vi "Tool-Response Time.vi"() -> ()   [LabVIEW 2015]
uses:
  <vilib>/measure/mamon.llb/Trigger Detection for 1 Channel.vi
  <vilib>/measure/NI_MAPro.lvlib
panel:
  in  "hysteresis":dbl=0.4 format="%.2f"
  out "Cursor Info.":string="[cursor_raw]\n X: 32.346,  Y: 0.9937658\n\n[cursor_filter]\n X: 30.672,  Y: 0.9937830"
  in  "Exit":bool=TRUE
  in  "Calcuration":bool
  out "trigger detected? 2":bool=TRUE caption="트리거 검출?"
  out "trigger detected?":bool=TRUE caption="트리거 검출?"
  in  "Trigger level (%)":dbl=50.0 min=0.0 max=100.0
  out "Delay_time(s)":dbl=1.6739999999999782
  out "Delta-Filter":dbl=0.00020839999999999748
  out "Delta-Raw":dbl=0.00011250000000007088
  out "Data Length":i32=1387
  out "Response Time Graph":cluster{dbl[], dbl[]}[](graph)
  in  "Data in (Raw & Filter)":string="Time (H:M:S) - Left Wing-C\tCDC Ratio Data - Left Wing-C\tTime (H:M:S) - Right Wing-A\tCDC Ratio Data - Right Wing-A\n29:01.379\t0.9937134\t29:01.379\t0.9937296\n29:01.407\t0.9937134\t29:01.407\t0.9937143\n29:01.434\t0.9937134\t29:01.434\t0.9937077\n29:01.462\t0.9937139\t29:01.462\t0.9937186\n29:01.490\t0.9937139\t29:01.490\t0.9937115\n29:01.518\t0.9937134\t29:01.518\t0.9936929\n29:01.547\t0.9937134\t29:01.547\t0.9936919\n29:01.575\t0.9937134\t29:01.575\t0.9937086\n29:01.629\t0.9937129\t29:01.629\t0.9937015\n29:01.657\t0.9937124\t29:01.657\t0.9936986\n29:01.685\t0.9937124\t29:01.685\t0.9936953\n29:01.714\t0.9937124\t29:01.714\t0.9936929\n29:01.742\t0.9937124\t29:01.742\t0.9937029\n29:01.770\t0.9937124\t29:01.770\t0.9937029\n29:01.798\t0.9937124\t29:01.798\t0.9937181\n29:01.826\t0.9937124\t29:01.826\t0.9937124\n29:01.851\t0.9937124\t29:01.851\t0.9937172\n29:01.880\t0.9937129\t29:01.880\t0.9937143\n29:01.908\t0.9937129\t29:01.908\t0.9937038\n29:01.936\t0.9937129\t29:01.936\t0.993711\n29:01.993\t0.9937134\t29:01.993\t0.9937177\n29:02.021\t0.9937134\t29:02.021\t0.993711\n29:02.049\t0.9937139\t29:02.049\t0.9937196\n29:02.075\t0.9937139\t29:02.075\t0.9937091\n29:02.103\t0.9937139\t29:02.103\t0.9936996\n29:02.131\t0.9937139\t29:02.131\t0.9937124\n29:02.159\t0.9937143\t29:02.159\t0.9937325\n29:02.188\t0.9937148\t29:02.188\t0.9937649\n29:02.217\t0.9937153\t29:02.217\t0.9937749\n29:02.245\t0.9937162\t29:02.245\t0.9937549\n29:02.272\t0.9937167\t29:02.272\t0.9937334\n29:02.301\t0.9937167\t29:02.301\t0.9937248\n29:02.326\t0.9937167\t29:02.326\t0.993731\n29:02.383\t0.9937167\t29:02.383\t0.9937205\n29:02.411\t0.9937167\t29:02.411\t0.9937253\n29:02.439\t0.9937167\t29:02.439\t0.9937162\n29:02.467\t0.9937167\t29:02.467\t0.993752\n29:02.495\t0.9937172\t29:02.495\t0.9937534\n29:02.524\t0.9937177\t29:02.524\t0.9937453\n29:02.552\t0.9937181\t29:02.552\t0.9937339\n29:02.578\t0.9937186\t29:02.578\t0.9937229\n29:02.606\t0.9937186\t29:02.606\t0.9937358\n29:02.634\t0.9937191\t29:02.634\t0.9937229\n29:02.662\t0.9937191\t29:02.662\t0.9937229\n29:02.690\t0.9937191\t29:02.690\t0.99371\n29:02.719\t0.9937196\t29:02.719\t0.9937177\n29:02.746\t0.9937196\t29:02.746\t0.9937148\n29:02.800\t0.9937196\t29:02.800\t0.9937005\n29:02.828\t0.9937196\t29:02.828\t0.9937129\n29:02.856\t0.9937196\t29:02.856\t0.9937096\n29:02.884\t0.9937191\t29:02.884\t0.9937091\n29:02.913\t0.9937191\t29:02.913\t0.9937139\n29:02.941\t0.9937191\t29:02.941\t0.993711\n29:02.969\t0.9937186\t29:02.969\t0.9937096\n29:02.997\t0.9937181\t29:02.997\t0.9937139\n29:03.023\t0.9937181\t29:03.023\t0.9937115\n29:03.051\t0.9937181\t29:03.051\t0.9937291\n29:03.079\t0.9937181\t29:03.079\t0.9937205\n29:03.107\t0.9937181\t29:03.107\t0.9937215\n29:03.135\t0.9937177\t29:03.135\t0.9937215\n29:03.192\t0.9937177\t29:03.192\t0.9937048\n29:03.220\t0.9937177\t29:03.220\t0.9937034\n29:03.246\t0.9937181\t29:03.246\t0.9937143\n29:03.274\t0.9937181\t29:03.274\t0.9937062\n29:03.302\t0.9937181\t29:03.302\t0.9937143\n29:03.330\t0.9937177\t29:03.330\t0.9937215\n29:03.358\t0.9937177\t29:03.358\t0.9937115\n29:03.387\t0.9937177\t29:03.387\t0.9937158\n29:03.415\t0.9937177\t29:03.415\t0.9937129\n29:03.443\t0.9937177\t29:03.443\t0.9937119\n29:03.469\t0.9937172\t29:03.469\t0.9936972\n29:03.497\t0.9937172\t29:03.497\t0.9937191\n29:03.524\t0.9937172\t29:03.524\t0.9937143\n29:03.580\t0.9937172\t29:03.580\t0.9937081\n29:03.608\t0.9937172\t29:03.608\t0.9937201\n29:03.637\t0.9937172\t29:03.637\t0.9937119\n29:03.665\t0.9937177\t29:03.665\t0.9937205\n29:03.691\t0.9937177\t29:03.691\t0.9937263\n29:03.719\t0.9937177\t29:03.719\t0.9937286\n29:03.747\t0.9937177\t29:03.747\t0.9937148\n29:03.776\t0.9937177\t29:03.776\t0.9937086\n29:03.803\t0.9937177\t29:03.803\t0.9937119\n29:03.832\t0.9937177\t29:03.832\t0.9937191\n29:03.860\t0.9937177\t29:03.860\t0.9937072\n29:03.889\t0.9937177\t29:03.889\t0.9937062\n29:03.942\t0.9937177\t29:03.942\t0.9937305\n29:03.970\t0.9937177\t29:03.970\t0.9937258\n29:03.998\t0.9937177\t29:03.998\t0.9937167\n29:04.026\t0.9937177\t29:04.026\t0.9937081\n29:04.055\t0.9937177\t29:04.055\t0.9936981\n29:04.083\t0.9937177\t29:04.083\t0.9936967\n29:04.111\t0.9937172\t29:04.111\t0.9936976\n29:04.139\t0.9937172\t29:04.139\t0.993711\n29:04.165\t0.9937167\t29:04.165\t0.9937081\n29:04.193\t0.9937167\t29:04.193\t0.9937081\n29:04.221\t0.9937162\t29:04.221\t0.9937105\n29:04.250\t0.9937162\t29:04.250\t0.9937019\n29:04.278\t0.9937162\t29:04.278\t0.9937143\n29:04.306\t0.9937158\t29:04.306\t0.9937143\n29:04.362\t0.9937158\t29:04.362\t0.9936996\n29:04.388\t0.9937158\t29:04.388\t0.9937091\n29:04.416\t0.9937158\t29:04.416\t0.9937005\n29:04.444\t0.9937158\t29:04.444\t0.993721\n29:04.471\t0.9937162\t29:04.471\t0.9937358\n29:04.500\t0.9937167\t29:04.500\t0.9937267\n29:04.528\t0.9937167\t29:04.528\t0.9937253\n29:04.557\t0.9937172\t29:04.557\t0.9937258\n29:04.584\t0.9937172\t29:04.584\t0.9937234\n29:04.610\t0.9937177\t29:04.610\t0.9937077\n29:04.638\t0.9937177\t29:04.638\t0.9936996\n29:04.666\t0.9937172\t29:04.666\t0.9937\n29:04.695\t0.9937172\t29:04.695\t0.99369\n29:04.751\t0.9937167\t29:04.751\t0.9936943\n29:04.779\t0.9937167\t29:04.779\t0.9937\n29:04.807\t0.9937167\t29:04.807\t0.9937019\n29:04.833\t0.9937167\t29:04.833\t0.9937081\n29:04.861\t0.9937162\t29:04.861\t0.9937186\n29:04.889\t0.9937162\t29:04.889\t0.9937134\n29:04.918\t0.9937162\t29:04.918\t0.9937148\n29:04.946\t0.9937162\t29:04.946\t0.9937034\n29:04.974\t0.9937162\t29:04.974\t0.9937096\n29:05.002\t0.9937162\t29:05.002\t0.993721\n29:05.030\t0.9937162\t29:05.030\t0.9937263\n29:05.056\t0.9937162\t29:05.056\t0.9937272\n29:05.086\t0.9937162\t29:05.086\t0.9937425\n29:05.141\t0.9937158\t29:05.141\t0.993741\n29:05.169\t0.9937158\t29:05.169\t0.9937348\n29:05.197\t0.9937158\t29:05.197\t0.9937181\n29:05.225\t0.9937153\t29:05.225\t0.9937248\n29:05.254\t0.9937153\t29:05.254\t0.9937215\n29:05.279\t0.9937153\t29:05.279\t0.9937191\n29:05.307\t0.9937153\t29:05.307\t0.9937057\n29:05.335\t0.9937153\t29:05.335\t0.9937019\n29:05.364\t0.9937148\t29:05.364\t0.9937057\n29:05.392\t0.9937143\t29:05.392\t0.9936972\n29:05.420\t0.9937139\t29:05.420\t0.9937091\n29:05.447\t0.9937139\t29:05.447\t0.9937196\n29:05.476\t0.9937139\t29:05.476\t0.9937196\n29:05.529\t0.9937134\t29:05.529\t0.993722\n29:05.558\t0.9937134\t29:05.558\t0.9937091\n29:05.586\t0.9937134\t29:05.586\t0.9937148\n29:05.614\t0.9937134\t29:05.614\t0.9937296\n29:05.642\t0.9937134\t29:05.642\t0.9937162\n29:05.670\t0.9937134\t29:05.670\t0.9937143\n29:05.699\t0.9937134\t29:05.699\t0.9937124\n29:05.725\t0.9937134\t29:05.725\t0.9937148\n29:05.753\t0.9937134\t29:05.753\t0.9937115\n29:05.781\t0.9937134\t29:05.781\t0.9937081\n29:05.809\t0.9937134\t29:05.809\t0.9937096\n29:05.837\t0.9937134\t29:05.837\t0.9937139\n29:05.865\t0.9937134\t29:05.865\t0.9937186\n29:05.922\t0.9937139\t29:05.922\t0.9937162\n29:05.947\t0.9937139\t29:05.947\t0.9937229\n29:05.976\t0.9937134\t29:05.976\t0.9937034\n29:06.004\t0.9937134\t29:06.004\t0.99371\n29:06.032\t0.9937134\t29:06.032\t0.9937191\n29:06.060\t0.9937134\t29:06.060\t0.9937129\n29:06.088\t0.9937134\t29:06.088\t0.9937091\n29:06.117\t0.9937134\t29:06.117\t0.9937134\n29:06.145\t0.9937134\t29:06.145\t0.9937124\n29:06.173\t0.9937134\t29:06.173\t0.9937129\n29:06.199\t0.9937134\t29:06.199\t0.9937139\n29:06.227\t0.9937134\t29:06.227\t0.9937143\n29:06.254\t0.9937134\t29:06.254\t0.9937258\n29:06.311\t0.9937139\t29:06.311\t0.9937372\n29:06.339\t0.9937143\t29:06.339\t0.9937348\n29:06.368\t0.9937143\t29:06.368\t0.9937272\n29:06.396\t0.9937148\t29:06.396\t0.9937205\n29:06.421\t0.9937148\t29:06.421\t0.9937215\n29:06.449\t0.9937148\t29:06.449\t0.9937148\n29:06.477\t0.9937148\t29:06.477\t0.9937201\n29:06.505\t0.9937153\t29:06.505\t0.993731\n29:06.534\t0.9937153\t29:06.534\t0.9937167\n29:06.562\t0.9937153\t29:06.562\t0.9937057\n29:06.590\t0.9937153\t29:06.590\t0.9937181\n29:06.618\t0.9937148\t29:06.618\t0.9937158\n29:06.672\t0.9937148\t29:06.672\t0.9937129\n29:06.700\t0.9937148\t29:06.700\t0.9937105\n29:06.729\t0.9937148\t29:06.729\t0.9937077\n29:06.758\t0.9937148\t29:06.758\t0.9937067\n29:06.785\t0.9937148\t29:06.785\t0.9937086\n29:06.813\t0.9937148\t29:06.813\t0.9937057\n29:06.841\t0.9937148\t29:06.841\t0.9937239\n29:06.869\t0.9937143\t29:06.869\t0.993722\n29:06.895\t0.9937143\t29:06.895\t0.9937162\n29:06.923\t0.9937143\t29:06.923\t0.9937186\n29:06.951\t0.9937148\t29:06.951\t0.99371\n29:06.980\t0.9937148\t29:06.980\t0.9937253\n29:07.009\t0.9937148\t29:07.009\t0.9937282\n29:07.036\t0.9937153\t29:07.036\t0.9937105\n29:07.093\t0.9937148\t29:07.093\t0.99371\n29:07.118\t0.9937148\t29:07.118\t0.9936905\n29:07.147\t0.9937148\t29:07.147\t0.9936919\n29:07.175\t0.9937148\t29:07.175\t0.9936991\n29:07.203\t0.9937148\t29:07.203\t0.9937267\n29:07.230\t0.9937153\t29:07.230\t0.993763\n29:07.259\t0.9937158\t29:07.259\t0.9937725\n29:07.288\t0.9937162\t29:07.288\t0.9937325\n29:07.316\t0.9937167\t29:07.316\t0.9937167\n29:07.342\t0.9937167\t29:07.342\t0.9937167\n29:07.369\t0.9937162\t29:07.369\t0.9937201\n29:07.397\t0.9937162\t29:07.397\t0.9937234\n29:07.425\t0.9937162\t29:07.425\t0.9937253\n29:07.482\t0.9937162\t29:07.482\t0.9937224\n29:07.510\t0.9937162\t29:07.510\t0.9937363\n29:07.538\t0.9937167\t29:07.538\t0.9937496\n29:07.564\t0.9937172\t29:07.564\t0.9937444\n29:07.592\t0.9937177\t29:07.592\t0.9937158\n29:07.621\t0.9937177\t29:07.621\t0.993721\n29:07.650\t0.9937181\t29:07.650\t0.9937296\n29:07.677\t0.9937181\t29:07.677\t0.9937143\n29:07.705\t0.9937186\t29:07.705\t0.9937291\n29:07.733\t0.9937186\t29:07.733\t0.9937124\n29:07.761\t0.9937191\t29:07.761\t0.9937196\n29:07.790\t0.9937191\t29:07.790\t0.9937248\n29:07.816\t0.9937191\t29:07.816\t0.9937124\n29:07.872\t0.9937191\t29:07.872\t0.9937072\n29:07.900\t0.9937191\t29:07.900\t0.9937067\n29:07.928\t0.9937186\t29:07.928\t0.9937067\n29:07.957\t0.9937186\t29:07.957\t0.9937186\n29:07.985\t0.9937186\t29:07.985\t0.9937229\n29:08.013\t0.9937186\t29:08.013\t0.9937282\n29:08.039\t0.9937181\t29:08.039\t0.9937215\n29:08.067\t0.9937181\t29:08.067\t0.9937239\n29:08.095\t0.9937181\t29:08.095\t0.9937301\n29:08.123\t0.9937181\t29:08.123\t0.9937215\n29:08.152\t0.9937181\t29:08.152\t0.9937258\n29:08.179\t0.9937186\t29:08.179\t0.9937291\n29:08.207\t0.9937186\t29:08.207\t0.9937248\n29:08.235\t0.9937186\t29:08.235\t0.9937177\n29:08.289\t0.9937191\t29:08.289\t0.9937086\n29:08.317\t0.9937191\t29:08.317\t0.9936976\n29:08.346\t0.9937186\t29:08.346\t0.9937015\n29:08.374\t0.9937186\t29:08.374\t0.9936996\n29:08.402\t0.9937186\t29:08.402\t0.9936991\n29:08.430\t0.9937181\t29:08.430\t0.9936891\n29:08.459\t0.9937181\t29:08.459\t0.9936881\n29:08.487\t0.9937177\t29:08.487\t0.9936938\n29:08.513\t0.9937177\t29:08.513\t0.9936962\n29:08.541\t0.9937172\t29:08.541\t0.993711\n29:08.569\t0.9937172\t29:08.569\t0.9937086\n29:08.597\t0.9937172\t29:08.597\t0.9937005\n29:08.625\t0.9937172\t29:08.625\t0.9936967\n29:08.682\t0.9937172\t29:08.682\t0.9937\n29:08.710\t0.9937172\t29:08.710\t0.9937072\n29:08.736\t0.9937172\t29:08.736\t0.9937296\n29:08.764\t0.9937172\t29:08.764\t0.9937272\n29:08.792\t0.9937172\t29:08.792\t0.9937096\n29:08.820\t0.9937167\t29:08.820\t0.9937072\n29:08.848\t0.9937167\t29:08.848\t0.9936991\n29:08.876\t0.9937167\t29:08.876\t0.9937086\n29:08.905\t0.9937167\t29:08.905\t0.9936957\n29:08.935\t0.9937162\t29:08.935\t0.9936905\n29:08.959\t0.9937162\t29:08.959\t0.9936996\n29:08.987\t0.9937162\t29:08.987\t0.9937158\n29:09.014\t0.9937162\t29:09.014\t0.9937115\n29:09.071\t0.9937162\t29:09.071\t0.9937096\n29:09.100\t0.9937162\t29:09.100\t0.9937005\n29:09.128\t0.9937162\t29:09.128\t0.9937124\n29:09.156\t0.9937158\t29:09.156\t0.9937029\n29:09.182\t0.9937158\t29:09.182\t0.9937153\n29:09.209\t0.9937153\t29:09.209\t0.99371\n29:09.237\t0.9937153\t29:09.237\t0.9937091\n29:09.266\t0.9937148\t29:09.266\t0.9937067\n29:09.294\t0.9937148\t29:09.294\t0.9936981\n29:09.322\t0.9937143\t29:09.322\t0.9937143\n29:09.350\t0.9937143\t29:09.350\t0.9937038\n29:09.379\t0.9937143\t29:09.379\t0.9936948\n29:09.407\t0.9937139\t29:09.407\t0.9937048\n29:09.461\t0.9937139\t29:09.461\t0.9937086\n29:09.489\t0.9937139\t29:09.489\t0.9937286\n29:09.518\t0.9937139\t29:09.518\t0.9937358\n29:09.545\t0.9937143\t29:09.545\t0.9937272\n29:09.573\t0.9937143\t29:09.573\t0.9937305\n29:09.602\t0.9937148\t29:09.602\t0.993731\n29:09.630\t0.9937148\t29:09.630\t0.9937229\n29:09.656\t0.9937148\t29:09.656\t0.9937134\n29:09.684\t0.9937148\t29:09.684\t0.9937048\n29:09.712\t0.9937148\t29:09.712\t0.9937019\n29:09.740\t0.9937148\t29:09.740\t0.9937024\n29:09.769\t0.9937148\t29:09.769\t0.9937172\n29:09.797\t0.9937148\t29:09.797\t0.9937086\n29:09.824\t0.9937148\t29:09.824\t0.9937043\n29:09.879\t0.9937143\t29:09.879\t0.9937072\n29:09.906\t0.9937143\t29:09.906\t0.9937005\n29:09.934\t0.9937143\t29:09.934\t0.9937\n29:09.963\t0.9937139\t29:09.963\t0.9937048\n29:09.991\t0.9937139\t29:09.991\t0.9936962\n29:10.019\t0.9937139\t29:10.019\t0.9937067\n29:10.047\t0.9937143\t29:10.047\t0.9937196\n29:10.076\t0.9937143\t29:10.076\t0.9937305\n29:10.104\t0.9937148\t29:10.104\t0.9937291\n29:10.129\t0.9937143\t29:10.129\t0.9937334\n29:10.158\t0.9937143\t29:10.158\t0.9937344\n29:10.186\t0.9937139\t29:10.186\t0.9937305\n29:10.242\t0.9937139\t29:10.242\t0.9937129\n29:10.270\t0.9937139\t29:10.270\t0.9937205\n29:10.299\t0.9937139\t29:10.299\t0.9937267\n29:10.328\t0.9937143\t29:10.328\t0.9937286\n29:10.353\t0.9937139\t29:10.353\t0.9937072\n29:10.381\t0.9937139\t29:10.381\t0.9937038\n29:10.409\t0.9937134\t29:10.409\t0.9936914\n29:10.437\t0.9937129\t29:10.437\t0.9936924\n29:10.466\t0.9937124\t29:10.466\t0.9937029\n29:10.494\t0.9937124\t29:10.494\t0.9937267\n29:10.522\t0.9937124\t29:10.522\t0.9937129\n29:10.550\t0.9937124\t29:10.550\t0.9937062\n29:10.576\t0.9937124\t29:10.576\t0.9937077\n29:10.631\t0.9937119\t29:10.631\t0.9937077\n29:10.660\t0.9937119\t29:10.660\t0.9937282\n29:10.688\t0.9937119\t29:10.688\t0.993721\n29:10.716\t0.9937119\t29:10.716\t0.9937029\n29:10.744\t0.9937119\t29:10.744\t0.9937096\n29:10.772\t0.9937119\t29:10.772\t0.9937172\n29:10.798\t0.9937119\t29:10.798\t0.9937119\n29:10.827\t0.9937124\t29:10.827\t0.9937172\n29:10.854\t0.9937124\t29:10.854\t0.9937134\n29:10.882\t0.9937119\t29:10.882\t0.9937062\n29:10.911\t0.9937119\t29:10.911\t0.9937201\n29:10.939\t0.9937119\t29:10.939\t0.9937215\n29:10.967\t0.9937119\t29:10.967\t0.9937253\n29:10.995\t0.9937119\t29:10.995\t0.9937286\n29:11.049\t0.9937119\t29:11.049\t0.9937296\n29:11.077\t0.9937119\t29:11.077\t0.993732\n29:11.106\t0.9937119\t29:11.106\t0.9937243\n29:11.134\t0.9937119\t29:11.134\t0.9937067\n29:11.162\t0.9937119\t29:11.162\t0.9937124\n29:11.190\t0.9937119\t29:11.190\t0.9937119\n29:11.218\t0.9937119\t29:11.218\t0.9937167\n29:11.247\t0.9937119\t29:11.247\t0.9937139\n29:11.273\t0.9937119\t29:11.273\t0.9937215\n29:11.301\t0.9937124\t29:11.301\t0.9937191\n29:11.329\t0.9937124\t29:11.329\t0.9937348\n29:11.357\t0.9937134\t29:11.357\t0.9937363\n29:11.386\t0.9937134\t29:11.386\t0.9937282\n29:11.442\t0.9937139\t29:11.442\t0.9937181\n29:11.470\t0.9937143\t29:11.470\t0.9937229\n29:11.496\t0.9937143\t29:11.496\t0.9937067\n29:11.524\t0.9937143\t29:11.524\t0.993722\n29:11.553\t0.9937143\t29:11.553\t0.9937186\n29:11.581\t0.9937143\t29:11.581\t0.9937067\n29:11.609\t0.9937143\t29:11.609\t0.9936967\n29:11.637\t0.9937143\t29:11.637\t0.99371\n29:11.664\t0.9937143\t29:11.664\t0.9937129\n29:11.693\t0.9937143\t29:11.693\t0.9937053\n29:11.719\t0.9937143\t29:11.719\t0.9937077\n29:11.747\t0.9937139\t29:11.747\t0.9936962\n29:11.775\t0.9937139\t29:11.775\t0.9937005\n29:11.831\t0.9937143\t29:11.831\t0.9937153\n29:11.860\t0.9937143\t29:11.860\t0.99371\n29:11.888\t0.9937143\t29:11.888\t0.9937201\n29:11.916\t0.9937148\t29:11.916\t0.9937224\n29:11.944\t0.9937148\t29:11.944\t0.9937234\n29:11.970\t0.9937148\t29:11.970\t0.9937172\n29:11.999\t0.9937148\t29:11.999\t0.9937167\n29:12.026\t0.9937153\t29:12.026\t0.9937267\n29:12.054\t0.9937153\t29:12.054\t0.9937296\n29:12.083\t0.9937158\t29:12.083\t0.9937191\n29:12.112\t0.9937158\t29:12.112\t0.9937129\n29:12.140\t0.9937158\t29:12.140\t0.9937153\n29:12.167\t0.9937158\t29:12.167\t0.9936981\n29:12.221\t0.9937158\t29:12.221\t0.993722\n29:12.249\t0.9937158\t29:12.249\t0.9937487\n29:12.278\t0.9937162\t29:12.278\t0.9937663\n29:12.306\t0.9937172\t29:12.306\t0.993762\n29:12.334\t0.9937177\t29:12.334\t0.9937377\n29:12.362\t0.9937177\t29:12.362\t0.9937143\n29:12.390\t0.9937177\t29:12.390\t0.9937263\n29:12.419\t0.9937177\t29:12.419\t0.9937162\n29:12.444\t0.9937172\t29:12.444\t0.9937196\n29:12.473\t0.9937172\t29:12.473\t0.9937234\n29:12.501\t0.9937172\t29:12.501\t0.9937239\n29:12.529\t0.9937172\t29:12.529\t0.9937253\n29:12.558\t0.9937172\t29:12.558\t0.9937382\n29:12.613\t0.9937181\t29:12.613\t0.9937301\n29:12.641\t0.9937181\t29:12.641\t0.9937043\n29:12.667\t0.9937181\t29:12.667\t0.9937196\n29:12.695\t0.9937181\t29:12.695\t0.9937139\n29:12.723\t0.9937181\t29:12.723\t0.9937143\n29:12.751\t0.9937181\t29:12.751\t0.9937186\n29:12.779\t0.9937181\t29:12.779\t0.9937181\n29:12.807\t0.9937186\t29:12.807\t0.9937177\n29:12.835\t0.9937186\t29:12.835\t0.9937248\n29:12.864\t0.9937186\t29:12.864\t0.9937124\n29:12.890\t0.9937191\t29:12.890\t0.9937081\n29:12.918\t0.9937191\t29:12.918\t0.9937105\n29:12.946\t0.9937191\t29:12.946\t0.9937062\n29:13.002\t0.9937186\t29:13.002\t0.993722\n29:13.030\t0.9937186\t29:13.030\t0.9937229\n29:13.060\t0.9937186\t29:13.060\t0.9937263\n29:13.087\t0.9937186\t29:13.087\t0.9937215\n29:13.113\t0.9937181\t29:13.113\t0.9937277\n29:13.141\t0.9937186\t29:13.141\t0.9937224\n29:13.169\t0.9937186\t29:13.169\t0.9937253\n29:13.197\t0.9937186\t29:13.197\t0.993731\n29:13.225\t0.9937186\t29:13.225\t0.9937215\n29:13.253\t0.9937186\t29:13.253\t0.9937172\n29:13.282\t0.9937186\t29:13.282\t0.9937019\n29:13.310\t0.9937186\t29:13.310\t0.9937186\n29:13.336\t0.9937186\t29:13.336\t0.9937053\n29:13.392\t0.9937186\t29:13.392\t0.993722\n29:13.420\t0.9937186\t29:13.420\t0.9937024\n29:13.449\t0.9937186\t29:13.449\t0.9937024\n29:13.477\t0.9937186\t29:13.477\t0.9936938\n29:13.504\t0.9937181\t29:13.504\t0.993701\n29:13.532\t0.9937181\t29:13.532\t0.9936986\n29:13.560\t0.9937181\t29:13.560\t0.9937129\n29:13.586\t0.9937181\t29:13.586\t0.9937196\n29:13.614\t0.9937181\t29:13.614\t0.9937191\n29:13.643\t0.9937181\t29:13.643\t0.993701\n29:13.670\t0.9937181\t29:13.670\t0.9937148\n29:13.699\t0.9937181\t29:13.699\t0.9937158\n29:13.727\t0.9937181\t29:13.727\t0.9937057\n29:13.755\t0.9937181\t29:13.755\t0.9937072\n29:13.809\t0.9937181\t29:13.809\t0.9937201\n29:13.837\t0.9937181\t29:13.837\t0.9937196\n29:13.866\t0.9937181\t29:13.866\t0.9937115\n29:13.894\t0.9937181\t29:13.894\t0.9937196\n29:13.922\t0.9937181\t29:13.922\t0.9937072\n29:13.950\t0.9937177\t29:13.950\t0.9937034\n29:13.978\t0.9937177\t29:13.978\t0.9937096\n29:14.007\t0.9937172\t29:14.007\t0.9937124\n29:14.033\t0.9937172\t29:14.033\t0.9937148\n29:14.061\t0.9937172\t29:14.061\t0.9937153\n29:14.089\t0.9937172\t29:14.089\t0.9937015\n29:14.117\t0.9937172\t29:14.117\t0.9937015\n29:14.173\t0.9937167\t29:14.173\t0.9936895\n29:14.202\t0.9937167\t29:14.202\t0.9936986\n29:14.229\t0.9937162\t29:14.229\t0.9937015\n29:14.255\t0.9937158\t29:14.255\t0.993701\n29:14.283\t0.9937158\t29:14.283\t0.9936967\n29:14.311\t0.9937153\t29:14.311\t0.9936924\n29:14.340\t0.9937153\t29:14.340\t0.9937086\n29:14.368\t0.9937153\t29:14.368\t0.9937048\n29:14.396\t0.9937148\t29:14.396\t0.9937005\n29:14.424\t0.9937148\t29:14.424\t0.9936962\n29:14.453\t0.9937148\t29:14.453\t0.9936962\n29:14.481\t0.9937143\t29:14.481\t0.9936948\n29:14.508\t0.9937143\t29:14.508\t0.9937096\n29:14.535\t0.9937148\t29:14.535\t0.9937282\n29:14.591\t0.9937153\t29:14.591\t0.9937325\n29:14.619\t0.9937153\t29:14.619\t0.9937291\n29:14.647\t0.9937158\t29:14.647\t0.9937372\n29:14.675\t0.9937158\t29:14.675\t0.993731\n29:14.704\t0.9937162\t29:14.704\t0.9937201\n29:14.729\t0.9937162\t29:14.729\t0.99371\n29:14.758\t0.9937162\t29:14.758\t0.9937096\n29:14.786\t0.9937158\t29:14.786\t0.9937086\n29:14.814\t0.9937158\t29:14.814\t0.9937143\n29:14.842\t0.9937158\t29:14.842\t0.9937077\n29:14.870\t0.9937153\t29:14.870\t0.9937105\n29:14.898\t0.9937153\t29:14.898\t0.9937124\n29:14.926\t0.9937153\t29:14.926\t0.9937062\n29:14.981\t0.9937153\t29:14.981\t0.9937115\n29:15.009\t0.9937153\t29:15.009\t0.993701\n29:15.036\t0.9937148\t29:15.036\t0.9937081\n29:15.065\t0.9937153\t29:15.065\t0.993721\n29:15.092\t0.9937153\t29:15.092\t0.9937258\n29:15.121\t0.9937158\t29:15.121\t0.9937267\n29:15.149\t0.9937158\t29:15.149\t0.993742\n29:15.175\t0.9937153\t29:15.175\t0.993742\n29:15.203\t0.9937153\t29:15.203\t0.9937472\n29:15.231\t0.9937153\t29:15.231\t0.9937429\n29:15.259\t0.9937153\t29:15.259\t0.9937296\n29:15.287\t0.9937153\t29:15.287\t0.9937243\n29:15.316\t0.9937153\t29:15.316\t0.9937243\n29:15.372\t0.9937153\t29:15.372\t0.9937215\n29:15.398\t0.9937153\t29:15.398\t0.9937029\n29:15.426\t0.9937153\t29:15.426\t0.9937077\n29:15.454\t0.9937148\t29:15.454\t0.9936976\n29:15.483\t0.9937143\t29:15.483\t0.993701\n29:15.511\t0.9937139\t29:15.511\t0.9937158\n29:15.539\t0.9937143\t29:15.539\t0.9937358\n29:15.568\t0.9937143\t29:15.568\t0.9937191\n29:15.596\t0.9937143\t29:15.596\t0.9937224\n29:15.624\t0.9937143\t29:15.624\t0.9937067\n29:15.650\t0.9937143\t29:15.650\t0.993701\n29:15.678\t0.9937143\t29:15.678\t0.9937215\n29:15.706\t0.9937143\t29:15.706\t0.9937153\n29:15.762\t0.9937139\t29:15.762\t0.9937096\n29:15.791\t0.9937143\t29:15.791\t0.9937177\n29:15.819\t0.9937143\t29:15.819\t0.9937315\n29:15.847\t0.9937143\t29:15.847\t0.9937143\n29:15.872\t0.9937143\t29:15.872\t0.9937277\n29:15.900\t0.9937143\t29:15.900\t0.9937258\n29:15.929\t0.9937143\t29:15.929\t0.9937162\n29:15.957\t0.9937143\t29:15.957\t0.9937191\n29:15.986\t0.9937143\t29:15.986\t0.9937162\n29:16.013\t0.9937143\t29:16.013\t0.9937258\n29:16.042\t0.9937143\t29:16.042\t0.9937177\n29:16.070\t0.9937143\t29:16.070\t0.9937105\n29:16.098\t0.9937139\t29:16.098\t0.9937177\n29:16.152\t0.9937139\t29:16.152\t0.9937038\n29:16.180\t0.9937139\t29:16.180\t0.9937\n29:16.208\t0.9937134\t29:16.208\t0.9936943\n29:16.236\t0.9937134\t29:16.236\t0.9936934\n29:16.264\t0.9937134\t29:16.264\t0.993701\n29:16.292\t0.9937129\t29:16.292\t0.9936948\n29:16.321\t0.9937129\t29:16.321\t0.9937143\n29:16.348\t0.9937134\t29:16.348\t0.9937315\n29:16.376\t0.9937134\t29:16.376\t0.9937296\n29:16.403\t0.9937139\t29:16.403\t0.9937382\n29:16.431\t0.9937139\t29:16.431\t0.9937248\n29:16.460\t0.9937143\t29:16.460\t0.9937243\n29:16.488\t0.9937143\t29:16.488\t0.9937286\n29:16.516\t0.9937143\t29:16.516\t0.9937239\n29:16.570\t0.9937148\t29:16.570\t0.9937253\n29:16.598\t0.9937148\t29:16.598\t0.9937177\n29:16.628\t0.9937148\t29:16.628\t0.9937062\n29:16.654\t0.9937148\t29:16.654\t0.9937024\n29:16.683\t0.9937143\t29:16.683\t0.9937162\n29:16.710\t0.9937143\t29:16.710\t0.99371\n29:16.738\t0.9937143\t29:16.738\t0.9937158\n29:16.767\t0.9937143\t29:16.767\t0.9937096\n29:16.796\t0.9937143\t29:16.796\t0.9937029\n29:16.820\t0.9937139\t29:16.820\t0.9937115\n29:16.849\t0.9937143\t29:16.849\t0.9937148\n29:16.877\t0.9937143\t29:16.877\t0.9937077\n29:16.906\t0.9937143\t29:16.906\t0.9937105\n29:16.961\t0.9937143\t29:16.961\t0.9937229\n29:16.989\t0.9937143\t29:16.989\t0.9937191\n29:17.018\t0.9937143\t29:17.018\t0.9937038\n29:17.044\t0.9937143\t29:17.044\t0.9937177\n29:17.072\t0.9937148\t29:17.072\t0.9937239\n29:17.100\t0.9937148\t29:17.100\t0.9937201\n29:17.128\t0.9937153\t29:17.128\t0.9937072\n29:17.156\t0.9937153\t29:17.156\t0.9937143\n29:17.184\t0.9937153\t29:17.184\t0.9937139\n29:17.213\t0.9937153\t29:17.213\t0.9937005\n29:17.241\t0.9937158\t29:17.241\t0.9937124\n29:17.267\t0.9937158\t29:17.267\t0.9937315\n29:17.296\t0.9937162\t29:17.296\t0.9937806\n29:17.351\t0.9937177\t29:17.351\t0.9937696\n29:17.379\t0.9937181\t29:17.379\t0.9937415\n29:17.407\t0.9937186\t29:17.407\t0.9937425\n29:17.436\t0.9937186\t29:17.436\t0.9937353\n29:17.464\t0.9937186\t29:17.464\t0.9937239\n29:17.490\t0.9937186\t29:17.490\t0.9937267\n29:17.518\t0.9937186\t29:17.518\t0.9937267\n29:17.546\t0.9937186\t29:17.546\t0.9937162\n29:17.574\t0.9937186\t29:17.574\t0.9937401\n29:17.602\t0.9937186\t29:17.602\t0.9937449\n29:17.630\t0.9937191\t29:17.630\t0.9937372\n29:17.659\t0.9937196\t29:17.659\t0.9937277\n29:17.686\t0.9937196\t29:17.686\t0.9937129\n29:17.740\t0.9937196\t29:17.740\t0.9937124\n29:17.769\t0.9937196\t29:17.769\t0.9937191\n29:17.796\t0.9937196\t29:17.796\t0.9937096\n29:17.826\t0.9937196\t29:17.826\t0.9937153\n29:17.853\t0.9937196\t29:17.853\t0.9937162\n29:17.881\t0.9937196\t29:17.881\t0.9937186\n29:17.909\t0.9937196\t29:17.909\t0.9937015\n29:17.936\t0.9937196\t29:17.936\t0.9937081\n29:17.963\t0.9937196\t29:17.963\t0.9937105\n29:17.991\t0.9937196\t29:17.991\t0.9937053\n29:18.019\t0.9937191\t29:18.019\t0.9937153\n29:18.048\t0.9937191\t29:18.048\t0.9937148\n29:18.076\t0.9937186\t29:18.076\t0.9937134\n29:18.132\t0.9937181\t29:18.132\t0.9937167\n29:18.160\t0.9937181\t29:18.160\t0.9937296\n29:18.186\t0.9937181\t29:18.186\t0.9937124\n29:18.214\t0.9937181\t29:18.214\t0.9937239\n29:18.242\t0.9937181\t29:18.242\t0.9937239\n29:18.271\t0.9937181\t29:18.271\t0.9937153\n29:18.299\t0.9937181\t29:18.299\t0.99371\n29:18.327\t0.9937181\t29:18.327\t0.9937057\n29:18.356\t0.9937181\t29:18.356\t0.9937172\n29:18.384\t0.9937181\t29:18.384\t0.9937134\n29:18.409\t0.9937186\t29:18.409\t0.993731\n29:18.438\t0.9937186\t29:18.438\t0.9937348\n29:18.466\t0.9937181\t29:18.466\t0.9937148\n29:18.521\t0.9937181\t29:18.521\t0.9937224\n29:18.549\t0.9937186\t29:18.549\t0.9937258\n29:18.578\t0.9937186\t29:18.578\t0.9937234\n29:18.607\t0.9937186\t29:18.607\t0.9937353\n29:18.631\t0.9937191\t29:18.631\t0.9937468\n29:18.660\t0.9937191\t29:18.660\t0.9937444\n29:18.688\t0.9937196\t29:18.688\t0.9937272\n29:18.716\t0.9937196\t29:18.716\t0.9937482\n29:18.744\t0.9937201\t29:18.744\t0.993742\n29:18.773\t0.9937201\t29:18.773\t0.9937339\n29:18.801\t0.9937201\t29:18.801\t0.9937496\n29:18.829\t0.9937205\t29:18.829\t0.9937611\n29:18.856\t0.993721\t29:18.856\t0.9937544\n29:18.911\t0.9937215\t29:18.911\t0.9937372\n29:18.940\t0.9937215\t29:18.940\t0.993742\n29:18.968\t0.993722\t29:18.968\t0.9937329\n29:18.996\t0.993722\t29:18.996\t0.9937334\n29:19.024\t0.993722\t29:19.024\t0.993732\n29:19.052\t0.9937224\t29:19.052\t0.9937587\n29:19.081\t0.9937229\t29:19.081\t0.9937472\n29:19.107\t0.9937239\t29:19.107\t0.9937568\n29:19.135\t0.9937239\t29:19.135\t0.993751\n29:19.163\t0.9937243\t29:19.163\t0.9937482\n29:19.191\t0.9937248\t29:19.191\t0.993742\n29:19.219\t0.9937253\t29:19.219\t0.9937315\n29:19.249\t0.9937258\t29:19.249\t0.9937434\n29:19.276\t0.9937258\t29:19.276\t0.9937382\n29:19.329\t0.9937258\t29:19.329\t0.993731\n29:19.358\t0.9937258\t29:19.358\t0.9937296\n29:19.386\t0.9937258\t29:19.386\t0.9937296\n29:19.413\t0.9937258\t29:19.413\t0.9937334\n29:19.442\t0.9937263\t29:19.442\t0.9937329\n29:19.470\t0.9937263\t29:19.470\t0.9937382\n29:19.499\t0.9937263\t29:19.499\t0.9937444\n29:19.526\t0.9937267\t29:19.526\t0.9937401\n29:19.553\t0.9937272\t29:19.553\t0.9937644\n29:19.580\t0.9937277\t29:19.580\t0.9937806\n29:19.608\t0.9937282\t29:19.608\t0.9937768\n29:19.638\t0.9937291\t29:19.638\t0.9937701\n29:19.666\t0.9937296\t29:19.666\t0.9937634\n29:19.721\t0.9937305\t29:19.721\t0.9937572\n29:19.749\t0.993731\t29:19.749\t0.9937477\n29:19.776\t0.9937315\t29:19.776\t0.9937348\n29:19.804\t0.9937315\t29:19.804\t0.9937296\n29:19.832\t0.9937315\t29:19.832\t0.9937463\n29:19.860\t0.993732\t29:19.860\t0.9937458\n29:19.888\t0.9937325\t29:19.888\t0.9937468\n29:19.916\t0.9937325\t29:19.916\t0.9937477\n29:19.945\t0.9937329\t29:19.945\t0.9937544\n29:19.972\t0.9937334\t29:19.972\t0.9937596\n29:19.998\t0.9937339\t29:19.998\t0.9937592\n29:20.027\t0.9937344\t29:20.027\t0.993763\n29:20.055\t0.9937344\t29:20.055\t0.9937563\n29:20.111\t0.9937358\t29:20.111\t0.9937782\n29:20.139\t0.9937363\t29:20.139\t0.9937835\n29:20.168\t0.9937367\t29:20.168\t0.9937782\n29:20.196\t0.9937372\t29:20.196\t0.993782\n29:20.222\t0.9937372\t29:20.222\t0.9937825\n29:20.250\t0.9937372\t29:20.250\t0.9937863\n29:20.278\t0.9937377\t29:20.278\t0.9937873\n29:20.306\t0.9937377\t29:20.306\t0.9937625\n29:20.333\t0.9937382\t29:20.333\t0.9937701\n29:20.362\t0.9937387\t29:20.362\t0.9937744\n29:20.390\t0.9937391\t29:20.390\t0.993783\n29:20.419\t0.9937396\t29:20.419\t0.9937644\n29:20.448\t0.9937401\t29:20.448\t0.9937611\n29:20.501\t0.9937401\t29:20.501\t0.9937458\n29:20.528\t0.9937406\t29:20.528\t0.9937658\n29:20.558\t0.9937406\t29:20.558\t0.9937763\n29:20.586\t0.9937415\t29:20.586\t0.9937887\n29:20.613\t0.993742\t29:20.613\t0.9937792\n29:20.641\t0.9937425\t29:20.641\t0.9937706\n29:20.670\t0.9937429\t29:20.670\t0.9937592\n29:20.696\t0.9937434\t29:20.696\t0.9937673\n29:20.724\t0.9937439\t29:20.724\t0.993783\n29:20.752\t0.9937449\t29:20.752\t0.9937763\n29:20.780\t0.9937453\t29:20.780\t0.9937749\n29:20.808\t0.9937458\t29:20.808\t0.9937758\n29:20.837\t0.9937468\t29:20.837\t0.993782\n29:20.866\t0.9937472\t29:20.866\t0.9937825\n29:20.922\t0.9937487\t29:20.922\t0.9937735\n29:20.947\t0.9937491\t29:20.947\t0.9937673\n29:20.976\t0.9937496\t29:20.976\t0.9937758\n29:21.004\t0.9937501\t29:21.004\t0.9937854\n29:21.033\t0.993751\t29:21.033\t0.9937792\n29:21.060\t0.9937515\t29:21.060\t0.9937878\n29:21.088\t0.993752\t29:21.088\t0.9937797\n29:21.117\t0.9937525\t29:21.117\t0.9937773\n29:21.144\t0.9937534\t29:21.144\t0.9937797\n29:21.170\t0.9937539\t29:21.170\t0.9937763\n29:21.199\t0.9937544\t29:21.199\t0.9937663\n29:21.227\t0.9937549\t29:21.227\t0.9937654\n29:21.283\t0.9937558\t29:21.283\t0.9937677\n29:21.311\t0.9937563\t29:21.311\t0.9937744\n29:21.339\t0.9937568\t29:21.339\t0.9937725\n29:21.368\t0.9937572\t29:21.368\t0.993783\n29:21.396\t0.9937582\t29:21.396\t0.9937906\n29:21.421\t0.9937592\t29:21.421\t0.9938021\n29:21.450\t0.9937596\t29:21.450\t0.9938097\n29:21.478\t0.9937601\t29:21.478\t0.9937987\n29:21.506\t0.9937611\t29:21.506\t0.9937978\n29:21.534\t0.9937615\t29:21.534\t0.9938011\n29:21.562\t0.993762\t29:21.562\t0.9937887\n29:21.591\t0.993763\t29:21.591\t0.9938006\n29:21.619\t0.9937634\t29:21.619\t0.9938035\n29:21.646\t0.9937639\t29:21.646\t0.9937897\n29:21.701\t0.9937649\t29:21.701\t0.9937873\n29:21.731\t0.9937649\t29:21.731\t0.993794\n29:21.758\t0.9937654\t29:21.758\t0.993782\n29:21.786\t0.9937658\t29:21.786\t0.993783\n29:21.814\t0.9937663\t29:21.814\t0.9937778\n29:21.842\t0.9937663\t29:21.842\t0.9937692\n29:21.871\t0.9937668\t29:21.871\t0.9937901\n29:21.896\t0.9937677\t29:21.896\t0.9937892\n29:21.926\t0.9937677\t29:21.926\t0.9937797\n29:21.953\t0.9937682\t29:21.953\t0.9938025\n29:21.981\t0.9937687\t29:21.981\t0.993794\n29:22.009\t0.9937692\t29:22.009\t0.9938006\n29:22.039\t0.9937696\t29:22.039\t0.9937983\n29:22.066\t0.9937701\t29:22.066\t0.9937892\n29:22.120\t0.9937716\t29:22.120\t0.9938121\n29:22.148\t0.993772\t29:22.148\t0.9938002\n29:22.175\t0.9937725\t29:22.175\t0.9937906\n29:22.203\t0.9937735\t29:22.203\t0.9938064\n29:22.232\t0.9937739\t29:22.232\t0.993794\n29:22.260\t0.9937744\t29:22.260\t0.9937921\n29:22.289\t0.9937754\t29:22.289\t0.9937916\n29:22.316\t0.9937758\t29:22.316\t0.9938397\n29:22.346\t0.9937773\t29:22.346\t0.9938598\n29:22.371\t0.9937787\t29:22.371\t0.9938564\n29:22.399\t0.9937792\t29:22.399\t0.993835\n29:22.427\t0.9937801\t29:22.427\t0.9938121\n29:22.456\t0.9937806\t29:22.456\t0.9938154\n29:22.511\t0.9937811\t29:22.511\t0.9938092\n29:22.540\t0.9937816\t29:22.540\t0.9938068\n29:22.568\t0.993782\t29:22.568\t0.9938188\n29:22.594\t0.9937825\t29:22.594\t0.9938111\n29:22.622\t0.9937835\t29:22.622\t0.9938288\n29:22.650\t0.993784\t29:22.650\t0.9938426\n29:22.679\t0.9937849\t29:22.679\t0.993835\n29:22.707\t0.9937859\t29:22.707\t0.9938231\n29:22.736\t0.9937863\t29:22.736\t0.9938083\n29:22.763\t0.9937873\t29:22.763\t0.9938192\n29:22.791\t0.9937878\t29:22.791\t0.9938159\n29:22.820\t0.9937887\t29:22.820\t0.9938126\n29:22.846\t0.9937892\t29:22.846\t0.9938073\n29:22.903\t0.9937901\t29:22.903\t0.9938097\n29:22.930\t0.9937906\t29:22.930\t0.9938064\n29:22.958\t0.9937911\t29:22.958\t0.9937873\n29:22.987\t0.9937916\t29:22.987\t0.9937963\n29:23.015\t0.9937916\t29:23.015\t0.9937997\n29:23.043\t0.9937921\t29:23.043\t0.9938068\n29:23.069\t0.9937921\t29:23.069\t0.9938054\n29:23.097\t0.9937925\t29:23.097\t0.9938159\n29:23.124\t0.9937925\t29:23.124\t0.993814\n29:23.152\t0.993793\t29:23.152\t0.9938221\n29:23.181\t0.9937935\t29:23.181\t0.9938164\n29:23.209\t0.993794\t29:23.209\t0.9938202\n29:23.238\t0.9937944\t29:23.238\t0.9938188\n29:23.267\t0.9937949\t29:23.267\t0.9938207\n29:23.320\t0.9937959\t29:23.320\t0.9938159\n29:23.348\t0.9937963\t29:23.348\t0.9938064\n29:23.376\t0.9937963\t29:23.376\t0.9938116\n29:23.404\t0.9937973\t29:23.404\t0.9938092\n29:23.433\t0.9937978\t29:23.433\t0.9938097\n29:23.461\t0.9937983\t29:23.461\t0.9938159\n29:23.489\t0.9937983\t29:23.489\t0.9938068\n29:23.517\t0.9937987\t29:23.517\t0.9937954\n29:23.543\t0.9937987\t29:23.543\t0.993794\n29:23.571\t0.9937992\t29:23.571\t0.9938025\n29:23.600\t0.9937992\t29:23.600\t0.9938021\n29:23.628\t0.9937997\t29:23.628\t0.9937959\n29:23.656\t0.9938002\t29:23.656\t0.9938126\n29:23.712\t0.9938011\t29:23.712\t0.993814\n29:23.742\t0.9938016\t29:23.742\t0.9938221\n29:23.769\t0.9938016\t29:23.769\t0.9938188\n29:23.794\t0.9938021\t29:23.794\t0.9938064\n29:23.823\t0.9938025\t29:23.823\t0.9938231\n29:23.850\t0.993803\t29:23.850\t0.9938407\n29:23.878\t0.9938035\t29:23.878\t0.9938369\n29:23.906\t0.993804\t29:23.906\t0.9938226\n29:23.935\t0.9938045\t29:23.935\t0.9938126\n29:23.963\t0.9938049\t29:23.963\t0.9938207\n29:23.992\t0.9938049\t29:23.992\t0.9938154\n29:24.017\t0.9938054\t29:24.017\t0.9938035\n29:24.045\t0.9938054\t29:24.045\t0.9937983\n29:24.102\t0.9938059\t29:24.102\t0.9938235\n29:24.130\t0.9938068\t29:24.130\t0.9938188\n29:24.158\t0.9938068\t29:24.158\t0.9938054\n29:24.186\t0.9938073\t29:24.186\t0.9938059\n29:24.216\t0.9938078\t29:24.216\t0.9938006\n29:24.241\t0.9938083\t29:24.241\t0.9938073\n29:24.269\t0.9938083\t29:24.269\t0.9938097\n29:24.297\t0.9938087\t29:24.297\t0.9938178\n29:24.325\t0.9938087\t29:24.325\t0.9938207\n29:24.353\t0.9938087\t29:24.353\t0.9938159\n29:24.383\t0.9938087\t29:24.383\t0.9938045\n29:24.410\t0.9938092\t29:24.410\t0.9938164\n29:24.438\t0.9938092\t29:24.438\t0.9938111\n29:24.467\t0.9938092\t29:24.467\t0.9938083\n29:24.520\t0.9938092\t29:24.520\t0.9937959\n29:24.548\t0.9938092\t29:24.548\t0.9938021\n29:24.577\t0.9938097\t29:24.577\t0.9938006\n29:24.605\t0.9938097\t29:24.605\t0.9938211\n29:24.633\t0.9938102\t29:24.633\t0.9938288\n29:24.661\t0.9938107\t29:24.661\t0.9938192\n29:24.688\t0.9938107\t29:24.688\t0.9938211\n29:24.714\t0.9938111\t29:24.714\t0.9938273\n29:24.742\t0.9938116\t29:24.742\t0.9938269\n29:24.771\t0.9938121\t29:24.771\t0.9938068\n29:24.800\t0.9938121\t29:24.800\t0.9937997\n29:24.828\t0.9938126\t29:24.828\t0.9938054\n29:24.856\t0.9938126\t29:24.856\t0.9938016\n29:24.913\t0.9938126\t29:24.913\t0.9938126\n29:24.938\t0.993813\t29:24.938\t0.9938107\n29:24.966\t0.993813\t29:24.966\t0.9938111\n29:24.994\t0.993813\t29:24.994\t0.9938092\n29:25.022\t0.993813\t29:25.022\t0.9938059\n29:25.050\t0.993813\t29:25.050\t0.9938083\n29:25.079\t0.993813\t29:25.079\t0.9938068\n29:25.108\t0.993813\t29:25.108\t0.9938059\n29:25.136\t0.9938135\t29:25.136\t0.993824\n29:25.165\t0.993814\t29:25.165\t0.9938321\n29:25.189\t0.993814\t29:25.189\t0.9938264\n29:25.218\t0.9938145\t29:25.218\t0.9938359\n29:25.246\t0.993814\t29:25.246\t0.9938369\n29:25.302\t0.993814\t29:25.302\t0.9938388\n29:25.330\t0.993814\t29:25.330\t0.9938269\n29:25.358\t0.993814\t29:25.358\t0.9938145\n29:25.386\t0.993814\t29:25.386\t0.9938178\n29:25.412\t0.9938145\t29:25.412\t0.9938202\n29:25.441\t0.9938145\t29:25.441\t0.9938164\n29:25.469\t0.9938145\t29:25.469\t0.9938045\n29:25.498\t0.9938145\t29:25.498\t0.9938102\n29:25.525\t0.993814\t29:25.525\t0.9937987\n29:25.553\t0.9938135\t29:25.553\t0.9938087\n29:25.582\t0.9938135\t29:25.582\t0.9938107\n29:25.610\t0.9938135\t29:25.610\t0.9938374\n29:25.663\t0.9938135\t29:25.663\t0.9938283\n29:25.691\t0.9938135\t29:25.691\t0.9938259\n29:25.719\t0.9938135\t29:25.719\t0.9938135\n29:25.748\t0.993814\t29:25.748\t0.9938221\n29:25.775\t0.993814\t29:25.775\t0.9938226\n29:25.805\t0.993814\t29:25.805\t0.9938226\n29:25.833\t0.9938145\t29:25.833\t0.9938178\n29:25.860\t0.9938145\t29:25.860\t0.9938231\n29:25.886\t0.9938149\t29:25.886\t0.9938235\n29:25.914\t0.9938149\t29:25.914\t0.9938169\n29:25.942\t0.9938149\t29:25.942\t0.9938211\n29:25.971\t0.9938154\t29:25.971\t0.9938207\n29:26.000\t0.9938154\t29:26.000\t0.9938102\n29:26.027\t0.9938154\t29:26.027\t0.9938278\n29:26.055\t0.9938154\t29:26.055\t0.9938102\n29:26.109\t0.9938154\t29:26.109\t0.9938121\n29:26.137\t0.9938154\t29:26.137\t0.9938073\n29:26.166\t0.9938149\t29:26.166\t0.9938083\n29:26.194\t0.9938149\t29:26.194\t0.9938226\n29:26.222\t0.9938154\t29:26.222\t0.9938135\n29:26.251\t0.9938149\t29:26.251\t0.9938087\n29:26.278\t0.9938154\t29:26.278\t0.9938154\n29:26.307\t0.9938154\t29:26.307\t0.9938164\n29:26.333\t0.9938154\t29:26.333\t0.9938116\n29:26.361\t0.9938154\t29:26.361\t0.9938145\n29:26.389\t0.9938154\t29:26.389\t0.9938211\n29:26.417\t0.9938154\t29:26.417\t0.9938264\n29:26.472\t0.9938164\t29:26.472\t0.9938383\n29:26.502\t0.9938169\t29:26.502\t0.9938273\n29:26.529\t0.9938169\t29:26.529\t0.9938231\n29:26.555\t0.9938169\t29:26.555\t0.9938345\n29:26.584\t0.9938169\t29:26.584\t0.993824\n29:26.611\t0.9938169\t29:26.611\t0.9938154\n29:26.639\t0.9938173\t29:26.639\t0.9938321\n29:26.667\t0.9938173\t29:26.667\t0.993825\n29:26.696\t0.9938173\t29:26.696\t0.9938164\n29:26.724\t0.9938173\t29:26.724\t0.9938092\n29:26.752\t0.9938169\t29:26.752\t0.9938145\n29:26.781\t0.9938169\t29:26.781\t0.9938107\n29:26.806\t0.9938169\t29:26.806\t0.993814\n29:26.863\t0.9938164\t29:26.863\t0.9938064\n29:26.891\t0.9938164\t29:26.891\t0.9938149\n29:26.919\t0.9938164\t29:26.919\t0.9938164\n29:26.947\t0.9938169\t29:26.947\t0.9938111\n29:26.976\t0.9938169\t29:26.976\t0.9938188\n29:27.004\t0.9938169\t29:27.004\t0.9938183\n29:27.030\t0.9938169\t29:27.030\t0.9938331\n29:27.058\t0.9938169\t29:27.058\t0.9938269\n29:27.086\t0.9938173\t29:27.086\t0.9938207\n29:27.115\t0.9938173\t29:27.115\t0.9938107\n29:27.142\t0.9938173\t29:27.142\t0.9938307\n29:27.171\t0.9938178\t29:27.171\t0.9938226\n29:27.199\t0.9938178\t29:27.199\t0.9938107\n29:27.227\t0.9938178\t29:27.227\t0.9938116\n29:27.255\t0.9938173\t29:27.255\t0.9938126\n29:27.310\t0.9938173\t29:27.310\t0.9938049\n29:27.338\t0.9938173\t29:27.338\t0.9938183\n29:27.366\t0.9938178\t29:27.366\t0.9938564\n29:27.394\t0.9938183\t29:27.394\t0.9938922\n29:27.422\t0.9938192\t29:27.422\t0.9938664\n29:27.450\t0.9938197\t29:27.450\t0.9938383\n29:27.478\t0.9938202\t29:27.478\t0.9938378\n29:27.504\t0.9938202\t29:27.504\t0.9938374\n29:27.533\t0.9938207\t29:27.533\t0.9938254\n29:27.560\t0.9938207\t29:27.560\t0.9938307\n29:27.588\t0.9938207\t29:27.588\t0.9938207\n29:27.616\t0.9938207\t29:27.616\t0.9938154\n29:27.673\t0.9938207\t29:27.673\t0.9938474\n29:27.701\t0.9938211\t29:27.701\t0.9938502\n29:27.727\t0.9938216\t29:27.727\t0.9938369\n29:27.755\t0.9938216\t29:27.755\t0.9938083\n29:27.783\t0.9938216\t29:27.783\t0.9938221\n29:27.811\t0.9938221\t29:27.811\t0.9938202\n29:27.840\t0.9938221\t29:27.840\t0.9938192\n29:27.868\t0.9938221\t29:27.868\t0.9938059\n29:27.896\t0.9938221\t29:27.896\t0.9938116\n29:27.925\t0.9938221\t29:27.925\t0.9938149\n29:27.950\t0.9938221\t29:27.950\t0.9938178\n29:27.978\t0.9938221\t29:27.978\t0.9937935\n29:28.006\t0.9938221\t29:28.006\t0.9938002\n29:28.063\t0.9938216\t29:28.063\t0.9938092\n29:28.091\t0.9938216\t29:28.091\t0.9938188\n29:28.119\t0.9938216\t29:28.119\t0.9938245\n29:28.147\t0.9938211\t29:28.147\t0.9938149\n29:28.174\t0.9938211\t29:28.174\t0.9938197\n29:28.200\t0.9938211\t29:28.200\t0.9938216\n29:28.229\t0.9938211\t29:28.229\t0.9938264\n29:28.258\t0.9938211\t29:28.258\t0.9938312\n29:28.285\t0.9938211\t29:28.285\t0.9938354\n29:28.313\t0.9938211\t29:28.313\t0.9938312\n29:28.341\t0.9938211\t29:28.341\t0.9938226\n29:28.369\t0.9938211\t29:28.369\t0.9938087\n29:28.399\t0.9938211\t29:28.399\t0.993804\n29:28.452\t0.9938216\t29:28.452\t0.9938102\n29:28.480\t0.9938216\t29:28.480\t0.993813\n29:28.508\t0.9938216\t29:28.508\t0.9938259\n29:28.536\t0.9938216\t29:28.536\t0.9938073\n29:28.565\t0.9938211\t29:28.565\t0.993814\n29:28.593\t0.9938211\t29:28.593\t0.9938045\n29:28.621\t0.9938211\t29:28.621\t0.993804\n29:28.647\t0.9938207\t29:28.647\t0.9938049\n29:28.675\t0.9938207\t29:28.675\t0.9938169\n29:28.703\t0.9938207\t29:28.703\t0.9938154\n29:28.733\t0.9938207\t29:28.733\t0.993825\n29:28.760\t0.9938207\t29:28.760\t0.9938083\n29:28.788\t0.9938207\t29:28.788\t0.993825\n29:28.816\t0.9938207\t29:28.816\t0.9938188\n29:28.873\t0.9938202\t29:28.873\t0.993824\n29:28.898\t0.9938207\t29:28.898\t0.9938293\n29:28.927\t0.9938207\t29:28.927\t0.9938245\n29:28.955\t0.9938207\t29:28.955\t0.9938202\n29:28.984\t0.9938207\t29:28.984\t0.9938135\n29:29.011\t0.9938207\t29:29.011\t0.9938178\n29:29.039\t0.9938207\t29:29.039\t0.9938097\n29:29.068\t0.9938207\t29:29.068\t0.9938073\n29:29.097\t0.9938207\t29:29.097\t0.9938083\n29:29.122\t0.9938207\t29:29.122\t0.993824\n29:29.150\t0.9938207\t29:29.150\t0.9938202\n29:29.177\t0.9938207\t29:29.177\t0.9938126\n29:29.206\t0.9938207\t29:29.206\t0.9938107\n29:29.262\t0.9938207\t29:29.262\t0.9938073\n29:29.290\t0.9938202\t29:29.290\t0.9938025\n29:29.318\t0.9938202\t29:29.318\t0.9938092\n29:29.344\t0.9938197\t29:29.344\t0.9938021\n29:29.372\t0.9938197\t29:29.372\t0.993803\n29:29.400\t0.9938192\t29:29.400\t0.9938102\n29:29.428\t0.9938192\t29:29.428\t0.9938054\n29:29.457\t0.9938188\t29:29.457\t0.9937963\n29:29.485\t0.9938188\t29:29.485\t0.9938107\n29:29.513\t0.9938188\t29:29.513\t0.9938016\n29:29.541\t0.9938183\t29:29.541\t0.9938002\n29:29.567\t0.9938178\t29:29.567\t0.9938145\n29:29.595\t0.9938178\t29:29.595\t0.9938059\n29:29.651\t0.9938183\t29:29.651\t0.9938354\n29:29.679\t0.9938183\t29:29.679\t0.9938378\n29:29.708\t0.9938188\t29:29.708\t0.993835\n29:29.736\t0.9938188\t29:29.736\t0.9938321\n29:29.764\t0.9938188\t29:29.764\t0.993825\n29:29.794\t0.9938192\t29:29.794\t0.9938197\n29:29.819\t0.9938188\t29:29.819\t0.9938049\n29:29.848\t0.9938188\t29:29.848\t0.9938045\n29:29.875\t0.9938188\t29:29.875\t0.9937983\n29:29.903\t0.9938188\t29:29.903\t0.9938116\n29:29.931\t0.9938183\t29:29.931\t0.9938126\n29:29.960\t0.9938183\t29:29.960\t0.9938197\n29:29.988\t0.9938183\t29:29.988\t0.9938159\n29:30.016\t0.9938183\t29:30.016\t0.9938207\n29:30.070\t0.9938183\t29:30.070\t0.9938231\n29:30.097\t0.9938183\t29:30.097\t0.993824\n29:30.126\t0.9938183\t29:30.126\t0.9938169\n29:30.154\t0.9938183\t29:30.154\t0.9938135\n29:30.183\t0.9938188\t29:30.183\t0.9938397\n29:30.210\t0.9938192\t29:30.210\t0.9938455\n29:30.238\t0.9938192\t29:30.238\t0.9938412\n29:30.265\t0.9938192\t29:30.265\t0.9938488\n29:30.292\t0.9938192\t29:30.292\t0.9938483\n29:30.321\t0.9938188\t29:30.321\t0.9938431\n29:30.350\t0.9938188\t29:30.350\t0.9938431\n29:30.377\t0.9938188\t29:30.377\t0.9938188\n29:30.406\t0.9938183\t29:30.406\t0.9938297\n29:30.462\t0.9938183\t29:30.462\t0.993824\n29:30.490\t0.9938183\t29:30.490\t0.9938173\n29:30.516\t0.9938183\t29:30.516\t0.9938126\n29:30.545\t0.9938178\t29:30.545\t0.9938054\n29:30.572\t0.9938178\t29:30.572\t0.9938006\n29:30.601\t0.9938173\t29:30.601\t0.9938135\n29:30.629\t0.9938169\t29:30.629\t0.9938269\n29:30.657\t0.9938173\t29:30.657\t0.9938369\n29:30.685\t0.9938173\t29:30.685\t0.993824\n29:30.715\t0.9938173\t29:30.715\t0.9938197\n29:30.739\t0.9938173\t29:30.739\t0.993804\n29:30.768\t0.9938169\t29:30.768\t0.9938097\n29:30.796\t0.9938173\t29:30.796\t0.9938207\n29:30.851\t0.9938173\t29:30.851\t0.9938145\n29:30.880\t0.9938173\t29:30.880\t0.9938188\n29:30.908\t0.9938178\t29:30.908\t0.9938169\n29:30.936\t0.9938178\t29:30.936\t0.9938254\n29:30.964\t0.9938178\t29:30.964\t0.9938169\n29:30.990\t0.9938178\t29:30.990\t0.9938259\n29:31.018\t0.9938178\t29:31.018\t0.9938173\n29:31.046\t0.9938178\t29:31.046\t0.9938192\n29:31.075\t0.9938178\t29:31.075\t0.9938321\n29:31.103\t0.9938178\t29:31.103\t0.9938211\n29:31.132\t0.9938178\t29:31.132\t0.9938235\n29:31.159\t0.9938178\t29:31.159\t0.9938231\n29:31.187\t0.9938178\t29:31.187\t0.9938154\n29:31.241\t0.9938178\t29:31.241\t0.9938145\n29:31.269\t0.9938178\t29:31.269\t0.9938107\n29:31.298\t0.9938178\t29:31.298\t0.9938087\n29:31.326\t0.9938178\t29:31.326\t0.9938159\n29:31.355\t0.9938178\t29:31.355\t0.9938078\n29:31.382\t0.9938178\t29:31.382\t0.9938154\n29:31.411\t0.9938178\t29:31.411\t0.9938149\n29:31.436\t0.9938178\t29:31.436\t0.993825\n29:31.465\t0.9938178\t29:31.465\t0.9938426\n29:31.493\t0.9938183\t29:31.493\t0.9938383\n29:31.521\t0.9938188\t29:31.521\t0.9938512\n29:31.549\t0.9938188\t29:31.549\t0.9938345\n29:31.578\t0.9938192\t29:31.578\t0.993834\n29:31.607\t0.9938192\t29:31.607\t0.9938345\n29:31.662\t0.9938197\t29:31.662\t0.9938273\n29:31.688\t0.9938197\t29:31.688\t0.9938378\n29:31.715\t0.9938197\t29:31.715\t0.9938259\n29:31.744\t0.9938197\t29:31.744\t0.9938068\n29:31.772\t0.9938197\t29:31.772\t0.9938116\n29:31.800\t0.9938197\t29:31.800\t0.9938154\n29:31.828\t0.9938192\t29:31.828\t0.9938049\n29:31.857\t0.9938192\t29:31.857\t0.9938092\n29:31.885\t0.9938192\t29:31.885\t0.9938073\n29:31.910\t0.9938188\t29:31.910\t0.9938083\n29:31.938\t0.9938192\t29:31.938\t0.9938254\n29:31.967\t0.9938192\t29:31.967\t0.9938178\n29:31.995\t0.9938192\t29:31.995\t0.9937973\n29:32.051\t0.9938188\t29:32.051\t0.993783\n29:32.079\t0.9938183\t29:32.079\t0.9937782\n29:32.108\t0.9938178\t29:32.108\t0.9937596\n29:32.134\t0.9938173\t29:32.134\t0.9937472\n29:32.162\t0.9938169\t29:32.162\t0.9937611\n29:32.190\t0.9938169\t29:32.190\t0.9937525\n29:32.218\t0.9938159\t29:32.218\t0.9937434\n29:32.246\t0.9938154\t29:32.246\t0.9937224\n29:32.275\t0.9938145\t29:32.275\t0.9937325\n29:32.303\t0.9938135\t29:32.303\t0.9937229\n29:32.331\t0.9938126\t29:32.331\t0.9937072\n29:32.359\t0.9938121\t29:32.359\t0.993711\n29:32.385\t0.9938111\t29:32.385\t0.9937444\n29:32.441\t0.9938107\t29:32.441\t0.9937768\n29:32.469\t0.9938102\t29:32.469\t0.9937558\n29:32.498\t0.9938097\t29:32.498\t0.9937367\n29:32.526\t0.9938087\t29:32.526\t0.9937325\n29:32.554\t0.9938078\t29:32.554\t0.9937329\n29:32.583\t0.9938068\t29:32.583\t0.9937277\n29:32.608\t0.9938054\t29:32.608\t0.9937253\n29:32.636\t0.9938045\t29:32.636\t0.9937353\n29:32.665\t0.993804\t29:32.665\t0.99371\n29:32.693\t0.993803\t29:32.693\t0.993741\n29:32.721\t0.9938021\t29:32.721\t0.9937472\n29:32.749\t0.9938016\t29:32.749\t0.9937348\n29:32.777\t0.9938011\t29:32.777\t0.9937286\n29:32.805\t0.9938002\t29:32.805\t0.993722\n29:32.859\t0.9937983\t29:32.859\t0.9937215\n29:32.887\t0.9937978\t29:32.887\t0.9937172\n29:32.916\t0.9937968\t29:32.916\t0.9937205\n29:32.943\t0.9937959\t29:32.943\t0.9937234\n29:32.972\t0.9937949\t29:32.972\t0.993722\n29:33.000\t0.993794\t29:33.000\t0.993721\n29:33.028\t0.9937925\t29:33.028\t0.9937005\n29:33.056\t0.9937916\t29:33.056\t0.9937143\n29:33.082\t0.9937906\t29:33.082\t0.9937105\n29:33.110\t0.9937897\t29:33.110\t0.993711\n29:33.138\t0.9937882\t29:33.138\t0.9937096\n29:33.168\t0.9937873\t29:33.168\t0.9937177\n29:33.195\t0.9937859\t29:33.195\t0.9937129\n29:33.251\t0.9937835\t29:33.251\t0.9937201\n29:33.280\t0.9937825\t29:33.280\t0.9937229\n29:33.305\t0.9937816\t29:33.305\t0.993721\n29:33.334\t0.9937806\t29:33.334\t0.9937263\n29:33.362\t0.9937797\t29:33.362\t0.9937248\n29:33.390\t0.9937787\t29:33.390\t0.9937267\n29:33.418\t0.9937778\t29:33.418\t0.9937086\n29:33.447\t0.9937768\t29:33.447\t0.9937148\n29:33.475\t0.9937758\t29:33.475\t0.9937129\n29:33.503\t0.9937749\t29:33.503\t0.9937048\n29:33.531\t0.9937739\t29:33.531\t0.99371\n29:33.557\t0.9937725\t29:33.557\t0.9937086\n29:33.613\t0.9937706\t29:33.613\t0.9937015\n29:33.641\t0.9937696\t29:33.641\t0.9936957\n29:33.669\t0.9937682\t29:33.669\t0.9936976\n29:33.697\t0.9937673\t29:33.697\t0.9936919\n29:33.725\t0.9937658\t29:33.725\t0.993711\n29:33.754\t0.9937649\t29:33.754\t0.993722\n29:33.780\t0.9937639\t29:33.780\t0.9936976\n29:33.808\t0.9937625\t29:33.808\t0.9937\n29:33.836\t0.993762\t29:33.836\t0.9937124\n29:33.865\t0.9937606\t29:33.865\t0.9937\n29:33.892\t0.9937596\t29:33.892\t0.9937077\n29:33.921\t0.9937582\t29:33.921\t0.9937172\n29:33.949\t0.9937572\t29:33.949\t0.9937196\n29:33.978\t0.9937563\t29:33.978\t0.9937057\n29:34.005\t0.9937549\t29:34.005\t0.9937077\n29:34.059\t0.9937525\t29:34.059\t0.9937096\n29:34.088\t0.993752\t29:34.088\t0.9937053\n29:34.116\t0.9937506\t29:34.116\t0.9936986\n29:34.144\t0.9937496\t29:34.144\t0.9937005\n29:34.172\t0.9937487\t29:34.172\t0.9937234\n29:34.200\t0.9937477\t29:34.200\t0.9937139\n29:34.229\t0.9937463\t29:34.229\t0.9936986\n29:34.255\t0.9937453\t29:34.255\t0.9937015\n29:34.283\t0.9937439\t29:34.283\t0.9936924\n29:34.312\t0.9937434\t29:34.312\t0.9936962\n29:34.339\t0.993742\t29:34.339\t0.9936857\n29:34.367\t0.993741\t29:34.367\t0.9937086\n29:34.394\t0.9937396\t29:34.394\t0.9937038\n29:34.451\t0.9937363\t29:34.451\t0.9936957\n29:34.477\t0.9937348\t29:34.477\t0.9936948\n29:34.505\t0.9937339\t29:34.505\t0.9937043\n29:34.533\t0.9937329\t29:34.533\t0.9936962\n29:34.561\t0.9937315\t29:34.561\t0.9936838\n29:34.589\t0.9937301\t29:34.589\t0.9936905\n29:34.618\t0.9937286\t29:34.618\t0.9936996\n29:34.646\t0.9937277\t29:34.646\t0.9937019\n29:34.674\t0.9937267\t29:34.674\t0.9937272\n29:34.700\t0.9937258\t29:34.700\t0.9937334\n29:34.728\t0.9937248\t29:34.728\t0.9937201\n29:34.756\t0.9937243\t29:34.756\t0.9937248\n29:34.812\t0.9937224\t29:34.812\t0.9937272\n29:34.841\t0.9937215\t29:34.841\t0.993711\n29:34.869\t0.9937205\t29:34.869\t0.9936948\n29:34.897\t0.9937191\t29:34.897\t0.9936962\n29:34.923\t0.9937181\t29:34.923\t0.993691\n29:34.951\t0.9937172\t29:34.951\t0.9936972\n29:34.981\t0.9937167\t29:34.981\t0.9936962\n29:35.008\t0.9937158\t29:35.008\t0.9937038\n29:35.036\t0.9937153\t29:35.036\t0.9937053\n29:35.064\t0.9937148\t29:35.064\t0.9937072\n29:35.092\t0.9937143\t29:35.092\t0.9937162\n29:35.120\t0.9937139\t29:35.120\t0.9937038\n29:35.147\t0.9937139\t29:35.147\t0.9936996\n29:35.203\t0.9937134\t29:35.203\t0.9937043\n29:35.231\t0.9937134\t29:35.231\t0.9937296\n29:35.259\t0.9937139\t29:35.259\t0.993732\n29:35.288\t0.9937139\t29:35.288\t0.9937267\n29:35.315\t0.9937134\t29:35.315\t0.9937387\n29:35.343\t0.9937129\t29:35.343\t0.9937377\n29:35.372\t0.9937129\t29:35.372\t0.993731\n29:35.397\t0.9937124\t29:35.397\t0.9937243\n29:35.425\t0.9937124\t29:35.425\t0.9937096\n29:35.453\t0.9937124\t29:35.453\t0.9937139\n29:35.481\t0.9937119\t29:35.481\t0.9937186\n29:35.509\t0.9937119\t29:35.509\t0.9937124\n29:35.538\t0.9937119\t29:35.538\t0.9937048\n29:35.566\t0.9937119\t29:35.566\t0.9937053\n29:35.620\t0.993711\t29:35.620\t0.9937053\n29:35.649\t0.9937105\t29:35.649\t0.9937096\n29:35.676\t0.9937105\t29:35.676\t0.9937282\n29:35.704\t0.9937105\t29:35.704\t0.9937229\n29:35.733\t0.9937105\t29:35.733\t0.9937196\n29:35.761\t0.9937105\t29:35.761\t0.993722\n29:35.789\t0.9937105\t29:35.789\t0.9937057\n29:35.817\t0.9937105\t29:35.817\t0.9937158\n29:35.843\t0.9937105\t29:35.843\t0.993721\n29:35.871\t0.9937105\t29:35.871\t0.9937181\n29:35.900\t0.99371\t29:35.900\t0.9937167\n29:35.928\t0.99371\t29:35.928\t0.9937181\n29:35.956\t0.9937105\t29:35.956\t0.9937186\n29:36.012\t0.99371\t29:36.012\t0.9937086\n29:36.040\t0.99371\t29:36.040\t0.9937091\n29:36.066\t0.99371\t29:36.066\t0.9937024\n29:36.094\t0.99371\t29:36.094\t0.993722\n29:36.123\t0.99371\t29:36.123\t0.9937339\n29:36.152\t0.9937105\t29:36.152\t0.9937215\n29:36.179\t0.99371\t29:36.179\t0.9937267\n29:36.207\t0.99371\t29:36.207\t0.9937129\n29:36.235\t0.99371\t29:36.235\t0.9937134\n29:36.264\t0.99371\t29:36.264\t0.9937239\n29:36.292\t0.99371\t29:36.292\t0.9937191\n29:36.317\t0.9937096\t29:36.317\t0.9937081\n29:36.345\t0.9937096\t29:36.345\t0.9937081\n29:36.401\t0.9937096\t29:36.401\t0.9937115\n29:36.429\t0.9937096\t29:36.429\t0.9937134\n29:36.458\t0.9937096\t29:36.458\t0.9937224\n29:36.486\t0.99371\t29:36.486\t0.9937215\n29:36.515\t0.99371\t29:36.515\t0.9937329\n29:36.540\t0.9937105\t29:36.540\t0.9937401\n29:36.568\t0.993711\t29:36.568\t0.9937334\n29:36.597\t0.9937115\t29:36.597\t0.9937344\n29:36.625\t0.9937115\t29:36.625\t0.9937248\n29:36.653\t0.9937119\t29:36.653\t0.9937243\n29:36.681\t0.9937119\t29:36.681\t0.9937153\n29:36.709\t0.9937124\t29:36.709\t0.9937305\n29:36.737\t0.9937124\t29:36.737\t0.9937229\n29:36.791\t0.9937124\t29:36.791\t0.9937105\n29:36.819\t0.9937124\t29:36.819\t0.9937153\n29:36.849\t0.9937124\t29:36.849\t0.9937115\n29:36.876\t0.9937124\t29:36.876\t0.9936991\n29:36.904\t0.9937124\t29:36.904\t0.9936996\n29:36.933\t0.9937124\t29:36.933\t0.9936996\n29:36.960\t0.9937124\t29:36.960\t0.9937048\n29:36.986\t0.9937124\t29:36.986\t0.99371\n29:37.015\t0.9937124\t29:37.015\t0.9937105\n29:37.042\t0.9937124\t29:37.042\t0.9937077\n29:37.071\t0.9937124\t29:37.071\t0.9937224\n29:37.099\t0.9937124\t29:37.099\t0.9937229\n29:37.126\t0.9937129\t29:37.126\t0.9937129\n29:37.182\t0.9937129\t29:37.182\t0.9937086\n29:37.208\t0.9937134\t29:37.208\t0.9937277\n29:37.236\t0.9937134\t29:37.236\t0.9937239\n29:37.265\t0.9937139\t29:37.265\t0.9937282\n29:37.293\t0.9937139\t29:37.293\t0.9937172\n29:37.321\t0.9937139\t29:37.321\t0.9937191\n29:37.349\t0.9937143\t29:37.349\t0.9937024\n29:37.377\t0.9937143\t29:37.377\t0.9937062\n29:37.406\t0.9937143\t29:37.406\t0.9937186\n29:37.434\t0.9937148\t29:37.434\t0.9937572\n29:37.460\t0.9937158\t29:37.460\t0.9937901\n29:37.488\t0.9937167\t29:37.488\t0.9937644\n29:37.516\t0.9937172\t29:37.516\t0.9937544\n29:37.572\t0.9937177\t29:37.572\t0.9937329\n29:37.601\t0.9937177\t29:37.601\t0.993732\n29:37.629\t0.9937177\t29:37.629\t0.993731\n29:37.657\t0.9937177\t29:37.657\t0.9937282\n29:37.685\t0.9937181\t29:37.685\t0.9937296\n29:37.711\t0.9937181\t29:37.711\t0.9937377\n29:37.739\t0.9937181\t29:37.739\t0.993742\n29:37.768\t0.9937186\t29:37.768\t0.9937534\n29:37.796\t0.9937191\t29:37.796\t0.9937525\n29:37.823\t0.9937196\t29:37.823\t0.9937272\n29:37.853\t0.9937201\t29:37.853\t0.9937267\n29:37.881\t0.9937201\t29:37.881\t0.993722\n29:37.908\t0.9937205\t29:37.908\t0.9937162\n29:37.962\t0.9937205\t29:37.962\t0.993711\n29:37.990\t0.9937205\t29:37.990\t0.99371\n29:38.018\t0.9937205\t29:38.018\t0.9937162\n29:38.046\t0.993721\t29:38.046\t0.9937119\n29:38.075\t0.993721\t29:38.075\t0.9937038\n29:38.103\t0.993721\t29:38.103\t0.9937181\n29:38.131\t0.993721\t29:38.131\t0.9937124\n29:38.159\t0.9937205\t29:38.159\t0.9937148\n29:38.185\t0.9937205\t29:38.185\t0.9937243\n29:38.214\t0.9937205\t29:38.214\t0.9937286\n29:38.242\t0.9937205\t29:38.242\t0.993731\n29:38.270\t0.9937205\t29:38.270\t0.9937196\n29:38.298\t0.9937205\t29:38.298\t0.9937339\n29:38.326\t0.9937205\t29:38.326\t0.9937387\n29:38.355\t0.9937205\t29:38.355\t0.9937387\n29:38.411\t0.993721\t29:38.411\t0.9937325\n29:38.437\t0.993721\t29:38.437\t0.9937234\n29:38.465\t0.9937215\t29:38.465\t0.9937215\n29:38.493\t0.9937215\t29:38.493\t0.9937196\n29:38.521\t0.9937215\t29:38.521\t0.9937191\n29:38.550\t0.993722\t29:38.550\t0.9937081\n29:38.579\t0.9937215\t29:38.579\t0.9937215\n29:38.606\t0.9937215\t29:38.606\t0.9937048\n29:38.634\t0.9937215\t29:38.634\t0.9937067\n29:38.660\t0.993721\t29:38.660\t0.9936962\n29:38.688\t0.993721\t29:38.688\t0.9937029\n29:38.716\t0.993721\t29:38.716\t0.9937057\n29:38.773\t0.993721\t29:38.773\t0.9937158\n29:38.801\t0.993721\t29:38.801\t0.9937258\n29:38.829\t0.993721\t29:38.829\t0.9937043\n29:38.856\t0.993721\t29:38.856\t0.9937196\n29:38.882\t0.993721\t29:38.882\t0.9937081\n29:38.910\t0.993721\t29:38.910\t0.9937019\n29:38.938\t0.993721\t29:38.938\t0.9937091\n29:38.967\t0.993721\t29:38.967\t0.993731\n29:38.995\t0.993721\t29:38.995\t0.9937153\n29:39.023\t0.993721\t29:39.023\t0.9937143\n29:39.052\t0.993721\t29:39.052\t0.9937096\n29:39.080\t0.9937205\t29:39.080\t0.9937196\n29:39.108\t0.9937205\t29:39.108\t0.9937091\n29:39.162\t0.9937205\t29:39.162\t0.9936991\n29:39.190\t0.9937201\t29:39.190\t0.9937038\n29:39.218\t0.9937201\t29:39.218\t0.9937148\n29:39.246\t0.9937205\t29:39.246\t0.9937129\n29:39.275\t0.9937201\t29:39.275\t0.9937029\n29:39.303\t0.9937201\t29:39.303\t0.9937091\n29:39.331\t0.9937201\t29:39.331\t0.9936972\n29:39.357\t0.9937201\t29:39.357\t0.9936924\n29:39.385\t0.9937196\t29:39.385\t0.9937067\n29:39.413\t0.9937196\t29:39.413\t0.9937034\n29:39.441\t0.9937191\t29:39.441\t0.9937034\n29:39.470\t0.9937186\t29:39.470\t0.9937057\n29:39.498\t0.9937181\t29:39.498\t0.9936991\n29:39.526\t0.9937181\t29:39.526\t0.993691\n29:39.580\t0.9937172\t29:39.580\t0.9936967\n29:39.608\t0.9937172\t29:39.608\t0.9936943\n29:39.636\t0.9937167\t29:39.636\t0.9936948\n29:39.665\t0.9937167\t29:39.665\t0.9937115\n29:39.693\t0.9937167\t29:39.693\t0.9937229\n29:39.721\t0.9937172\t29:39.721\t0.9937429\n29:39.749\t0.9937172\t29:39.749\t0.9937472\n29:39.777\t0.9937177\t29:39.777\t0.9937391\n29:39.806\t0.9937181\t29:39.806\t0.9937334\n29:39.831\t0.9937181\t29:39.831\t0.9937344\n29:39.859\t0.9937186\t29:39.859\t0.9937234\n29:39.887\t0.9937186\t29:39.887\t0.9937153\n29:39.915\t0.9937186\t29:39.915\t0.9937086\n29:39.973\t0.9937186\t29:39.973\t0.9937201\n29:40.000\t0.9937186\t29:40.000\t0.993711\n29:40.029\t0.9937186\t29:40.029\t0.993711\n29:40.054\t0.9937181\t29:40.054\t0.9937124\n29:40.082\t0.9937186\t29:40.082\t0.9937091\n29:40.110\t0.9937181\t29:40.110\t0.9937134\n29:40.138\t0.9937181\t29:40.138\t0.9937153\n29:40.166\t0.9937181\t29:40.166\t0.9937167\n29:40.195\t0.9937181\t29:40.195\t0.9937139\n29:40.223\t0.9937181\t29:40.223\t0.9937167\n29:40.251\t0.9937181\t29:40.251\t0.9937382\n29:40.279\t0.9937186\t29:40.279\t0.9937458\n29:40.305\t0.9937191\t29:40.305\t0.9937425\n29:40.361\t0.9937191\t29:40.361\t0.993753\n29:40.390\t0.9937186\t29:40.390\t0.9937472\n29:40.418\t0.9937186\t29:40.418\t0.9937382\n29:40.446\t0.9937181\t29:40.446\t0.9937215\n29:40.474\t0.9937181\t29:40.474\t0.9937258\n29:40.503\t0.9937181\t29:40.503\t0.9937177\n29:40.528\t0.9937181\t29:40.528\t0.9937243\n29:40.557\t0.9937177\t29:40.557\t0.9937143\n29:40.585\t0.9937177\t29:40.585\t0.9937053\n29:40.613\t0.9937177\t29:40.613\t0.9937096\n29:40.641\t0.9937172\t29:40.641\t0.9936991\n29:40.668\t0.9937167\t29:40.668\t0.9937086\n29:40.698\t0.9937162\t29:40.698\t0.9937267\n29:40.726\t0.9937162\t29:40.726\t0.9937329\n29:40.779\t0.9937162\t29:40.779\t0.9937191\n29:40.807\t0.9937162\t29:40.807\t0.9937172\n29:40.835\t0.9937158\t29:40.835\t0.9937148\n29:40.863\t0.9937162\t29:40.863\t0.9937267\n29:40.892\t0.9937162\t29:40.892\t0.9937239\n29:40.920\t0.9937162\t29:40.920\t0.9937229\n29:40.948\t0.9937162\t29:40.948\t0.9937143\n29:40.977\t0.9937162\t29:40.977\t0.9937143\n29:41.002\t0.9937167\t29:41.002\t0.9937258\n29:41.031\t0.9937167\t29:41.031\t0.993721\n29:41.059\t0.9937167\t29:41.059\t0.9937296\n29:41.087\t0.9937167\t29:41.087\t0.9937172\n29:41.115\t0.9937167\t29:41.115\t0.9937224\n29:41.171\t0.9937167\t29:41.171\t0.9937277\n29:41.200\t0.9937167\t29:41.200\t0.9937344\n29:41.228\t0.9937167\t29:41.228\t0.9937286\n29:41.253\t0.9937167\t29:41.253\t0.9937215\n29:41.282\t0.9937167\t29:41.282\t0.993732\n29:41.310\t0.9937167\t29:41.310\t0.9937282\n29:41.338\t0.9937162\t29:41.338\t0.9937177\n29:41.366\t0.9937162\t29:41.366\t0.9937129\n29:41.395\t0.9937162\t29:41.395\t0.9937124\n29:41.423\t0.9937162\t29:41.423\t0.9937\n29:41.450\t0.9937162\t29:41.450\t0.9937119\n29:41.476\t0.9937162\t29:41.476\t0.9937153\n29:41.533\t0.9937162\t29:41.533\t0.9937315\n29:41.560\t0.9937167\t29:41.560\t0.9937296\n29:41.590\t0.9937172\t29:41.590\t0.9937406\n29:41.617\t0.9937172\t29:41.617\t0.993721\n29:41.645\t0.9937177\t29:41.645\t0.993721\n29:41.673\t0.9937177\t29:41.673\t0.9937286\n29:41.701\t0.9937177\t29:41.701\t0.9937229\n29:41.727\t0.9937177\t29:41.727\t0.9937258\n29:41.755\t0.9937181\t29:41.755\t0.9937277\n29:41.783\t0.9937181\t29:41.783\t0.9937201\n29:41.812\t0.9937181\t29:41.812\t0.9937015\n29:41.840\t0.9937181\t29:41.840\t0.9937043\n29:41.868\t0.9937177\t29:41.868\t0.9937129\n29:41.896\t0.9937177\t29:41.896\t0.9936967\n29:41.950\t0.9937172\t29:41.950\t0.99369\n29:41.978\t0.9937172\t29:41.978\t0.9936943\n29:42.006\t0.9937172\t29:42.006\t0.993701\n29:42.035\t0.9937172\t29:42.035\t0.9937057\n29:42.063\t0.9937172\t29:42.063\t0.9936996\n29:42.091\t0.9937172\t29:42.091\t0.9937105\n29:42.119\t0.9937172\t29:42.119\t0.9937148\n29:42.149\t0.9937172\t29:42.149\t0.9937258\n29:42.173\t0.9937177\t29:42.173\t0.9937253\n29:42.202\t0.9937177\t29:42.202\t0.9937072\n29:42.231\t0.9937177\t29:42.231\t0.9937172\n29:42.258\t0.9937177\t29:42.258\t0.9937234\n29:42.286\t0.9937181\t29:42.286\t0.9937243\n29:42.343\t0.9937186\t29:42.343\t0.9937186\n29:42.371\t0.9937186\t29:42.371\t0.9937072\n29:42.396\t0.9937186\t29:42.396\t0.9936991\n29:42.424\t0.9937186\t29:42.424\t0.9936991\n29:42.452\t0.9937191\t29:42.452\t0.9937277\n29:42.481\t0.9937191\t29:42.481\t0.9937549\n29:42.508\t0.9937201\t29:42.508\t0.9937606\n29:42.536\t0.9937205\t29:42.536\t0.9937501\n29:42.565\t0.993721\t29:42.565\t0.9937277\n29:42.593\t0.993721\t29:42.593\t0.9937181\n29:42.621\t0.993721\t29:42.621\t0.9937286\n29:42.648\t0.9937205\t29:42.648\t0.9937272\n29:42.675\t0.9937205\t29:42.675\t0.9937229\n29:42.731\t0.9937205\t29:42.731\t0.9937153\n29:42.760\t0.9937205\t29:42.760\t0.9937487\n29:42.788\t0.993721\t29:42.788\t0.9937463\n29:42.816\t0.993721\t29:42.816\t0.9937305\n29:42.844\t0.9937215\t29:42.844\t0.9937296\n29:42.870\t0.9937215\t29:42.870\t0.9937177\n29:42.899\t0.9937215\t29:42.899\t0.9937234\n29:42.926\t0.9937215\t29:42.926\t0.9937224\n29:42.955\t0.993722\t29:42.955\t0.9937296\n"
  # "Response Time Calculation"
  # "*Time Format - HH:MM:SS.000"
  # "* Paste Excel Data"
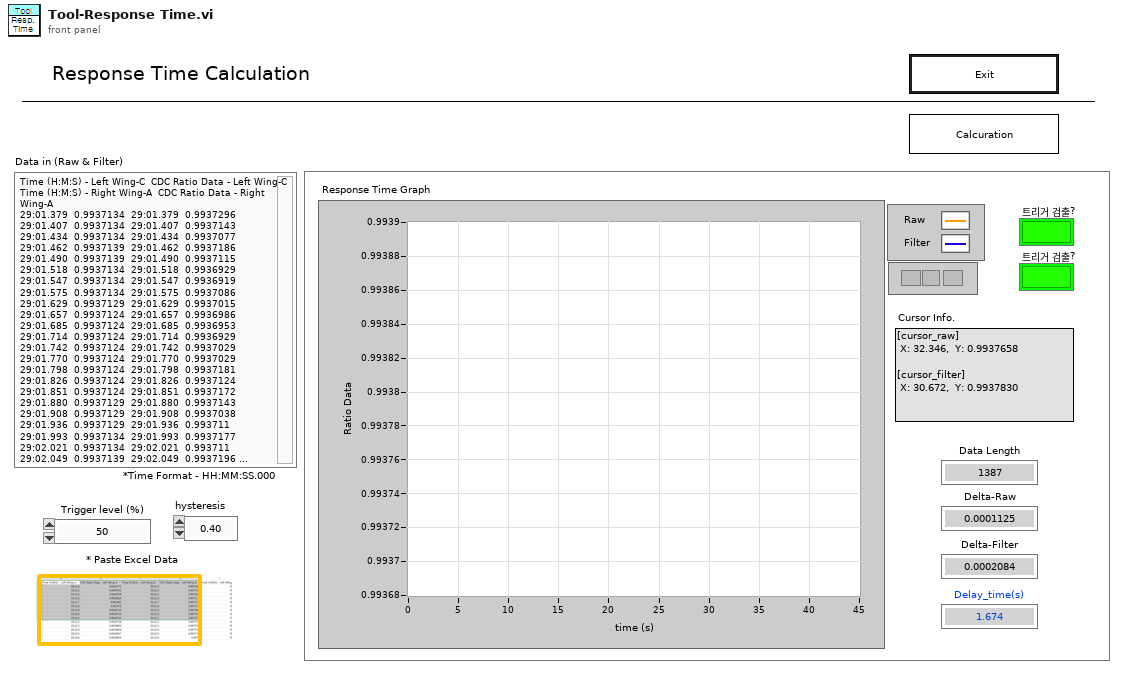
[diagram p1: front panel]
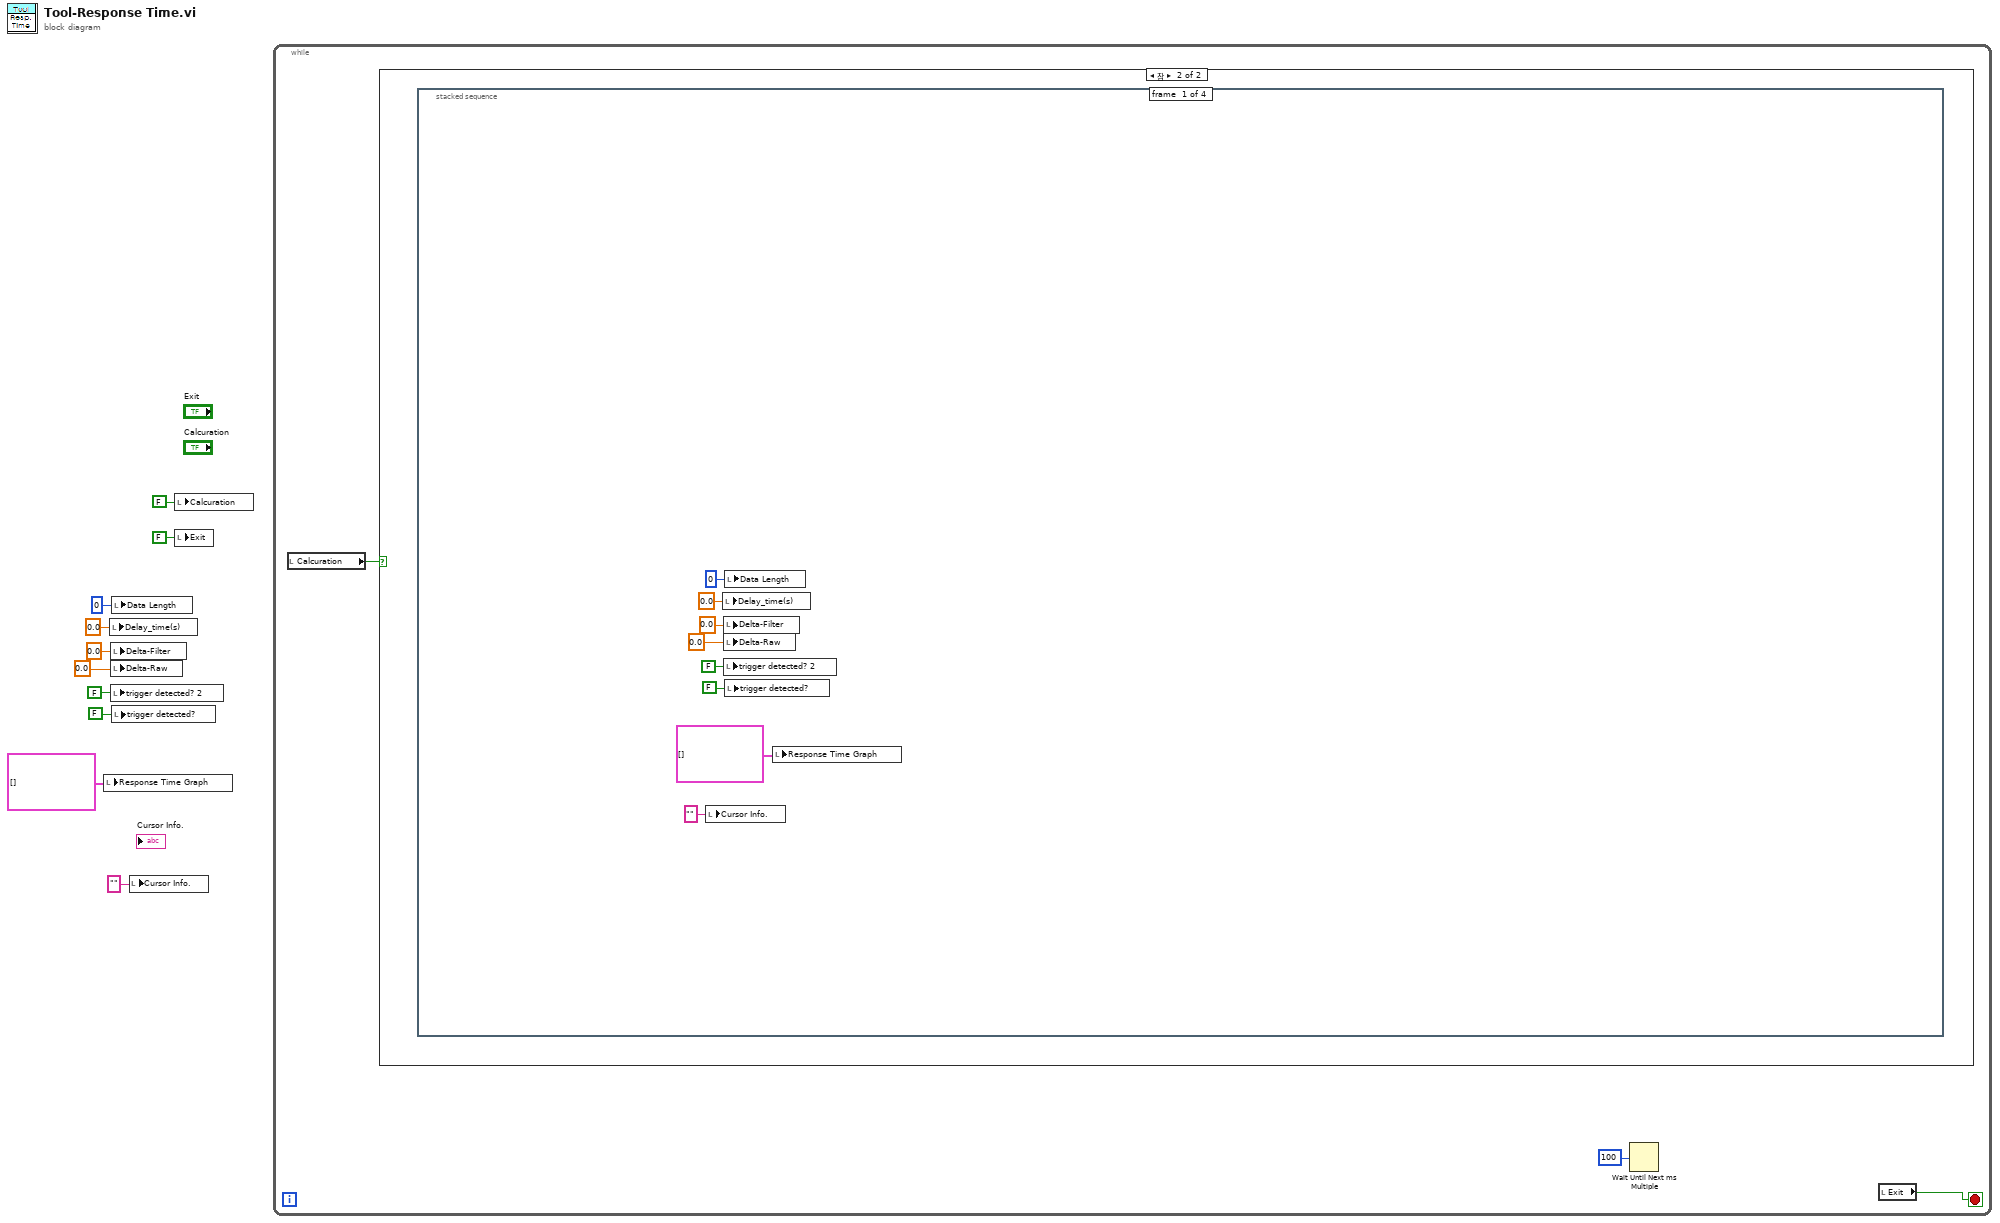
[diagram p0: block diagram]
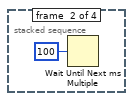
[diagram p3: hidden frame]
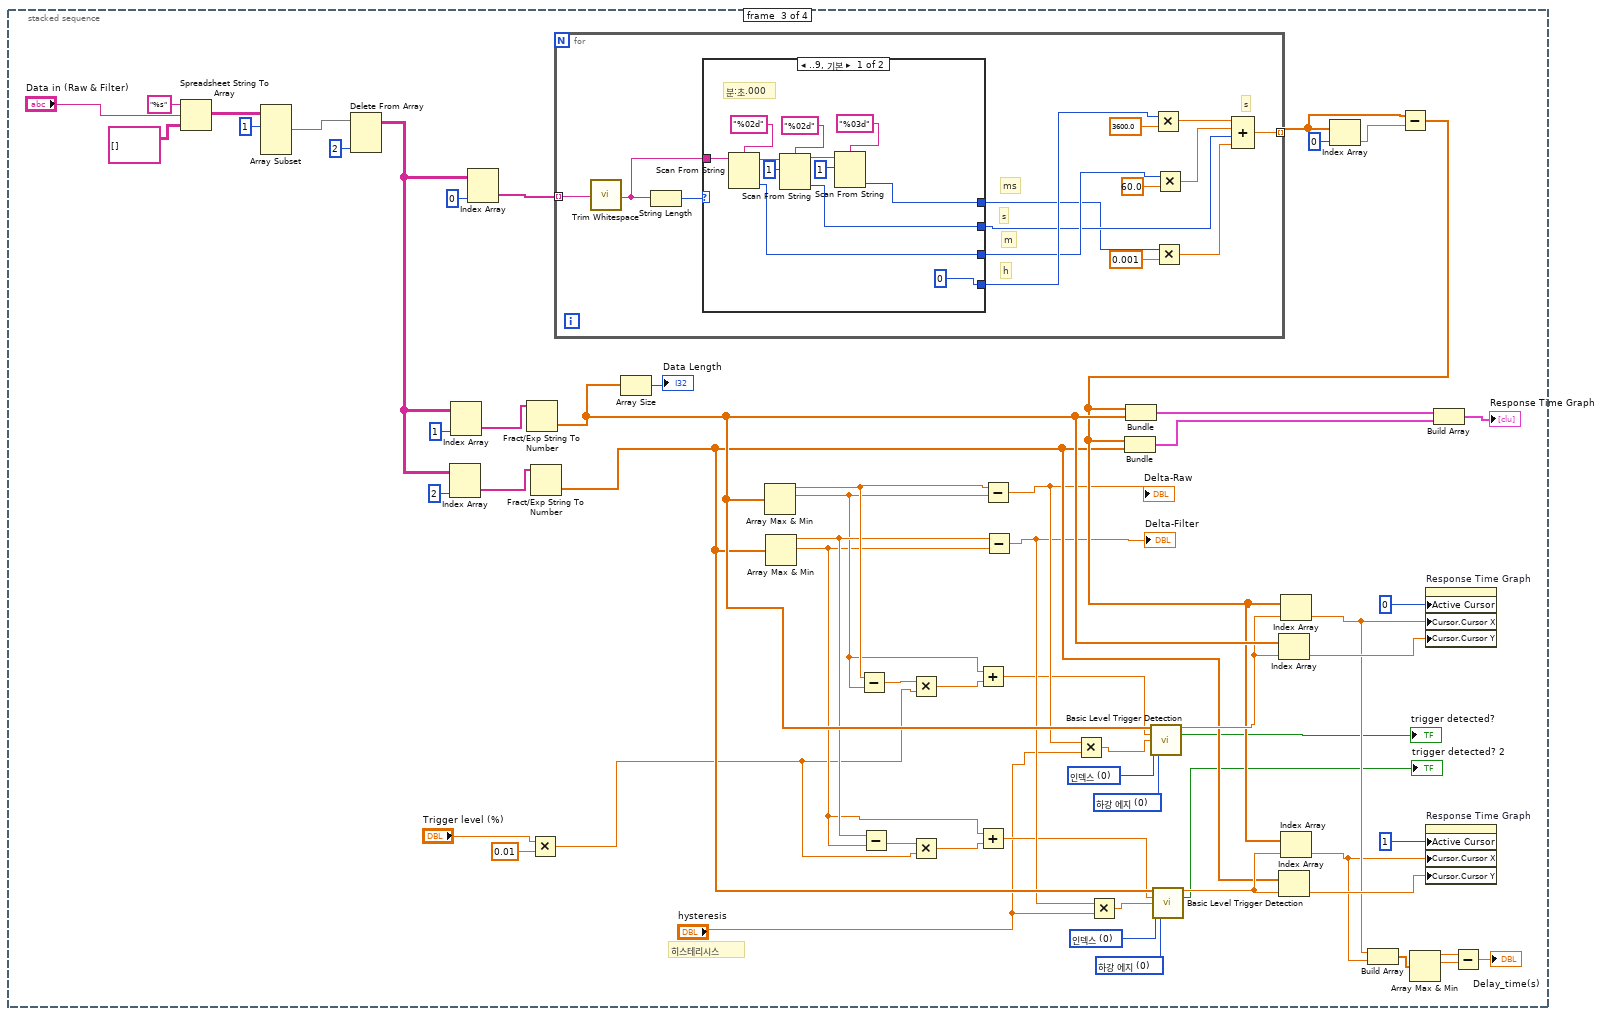
[diagram p4: hidden frame]
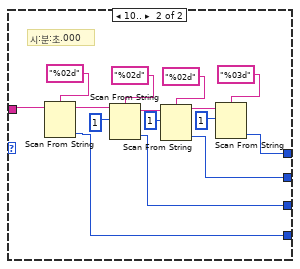
[diagram p5: hidden frame]
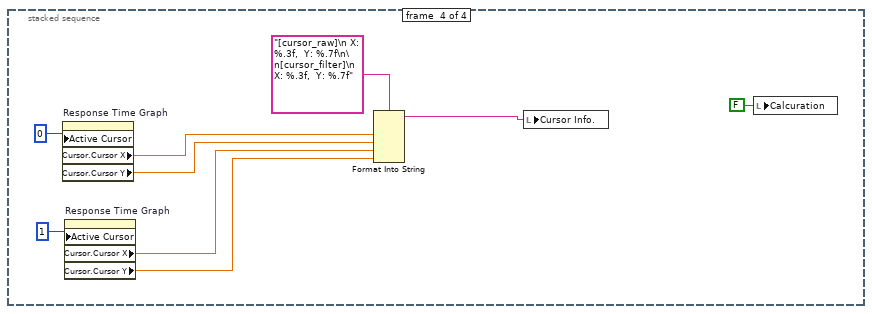
[diagram p6: hidden frame]
diagram:
  n1 = local write "Response Time Graph"(cluster{dbl[], dbl[]}[] [] ("Response Time Graph")) -> ()
  n2 = local write "Delay_time(s)"(0.0 ("Delay_time(s)")) -> ()
  n3 = local write "Delta-Filter"(0.0 ("Delta-Filter")) -> ()
  n4 = local write "Delta-Raw"(0.0 ("Delta-Raw")) -> ()
  n5 = local write "trigger detected? 2"(FALSE ("trigger detected? 2")) -> ()
  n6 = local write "Data Length"(0 ("Data Length")) -> ()
  n7 = local write "trigger detected?"(FALSE ("trigger detected?")) -> ()
  n8 = local write "Cursor Info."("" ("Cursor Info.")) -> ()
  n9 = local write "Calcuration"(FALSE ("Calcuration")) -> ()
  n10 = local write "Exit"(FALSE ("Exit")) -> ()
  n11 = while {
    stop <- w12 stop-if-true
    n12 = local read "Calcuration"() -> (w13:bool)
    n13 = case shown="참" w13 {
      frame False {
      }
      frame True {
        n14 = stacked-sequence {
          frame #0 {
            n15 = local write "Cursor Info."("" ("Cursor Info.")) -> ()
            n16 = local write "Delay_time(s)"(0.0 ("Delay_time(s)")) -> ()
            n17 = local write "Delta-Filter"(0.0 ("Delta-Filter")) -> ()
            n18 = local write "Delta-Raw"(0.0 ("Delta-Raw")) -> ()
            n19 = local write "trigger detected? 2"(FALSE ("trigger detected? 2")) -> ()
            n20 = local write "Data Length"(0 ("Data Length")) -> ()
            n21 = local write "trigger detected?"(FALSE ("trigger detected?")) -> ()
            n22 = local write "Response Time Graph"(cluster{dbl[], dbl[]}[] [] ("Response Time Graph")) -> ()
          }
          frame #1 {
            n23 = Wait Until Next ms Multiple(millisecond multiple=u32 100 ("ms 배수")) -> ()  [unwired: 1 out]
          }
          frame #2 {
            w54 = u16 0 items=["인덱스", "시간"] ("location mode")
            w53 = u16 0 items=["하강 에지", "상승 에지"] ("trigger slope")
            w59 = u16 0 items=["인덱스", "시간"] ("location mode")
            w60 = u16 0 items=["하강 에지", "상승 에지"] ("trigger slope")
            # "히스테리시스"
            n24 = Spreadsheet String To Array(format string="%s" ("포맷 문자열"), spreadsheet string="Data in (Raw & Filter)", array type (2D Dbl)=string[][] [] ("배열 타입(2D Dbl)")) -> (array=w79:string[][])  [unwired: 1 in]
            n25 = Array Subset(array=w79, index (row)=1 ("인덱스")) -> (w77:string[][])  [unwired: 3 in]
            n26 = Delete From Array(array=w77, index (col)=2 ("비활성화된 인덱스 (열)")) -> (array with subset deleted=w72:string[][])  [unwired: 2 in, 1 out]
            n27 = Index Array(array=w72, index (col)=2 ("비활성화된 인덱스 (열)")) -> (element=w69:string[])  [unwired: 1 in]
            n28 = Index Array(array=w72, index (col)=1 ("비활성화된 인덱스 (열)")) -> (element=w70:string[])  [unwired: 1 in]
            n29 = Index Array(array=w72, index (col)=0 ("비활성화된 인덱스 (열)")) -> (element=w71:string[])  [unwired: 1 in]
            n30 = Fract/Exp String To Number(string=w70) -> (number=w58:dbl[])  [unwired: 3 in, 1 out]
            n31 = Multiply(x="Trigger level (%)", y=0.01) -> (x*y=w25:dbl)
            n32 = Fract/Exp String To Number(string=w69) -> (number=w47:dbl[])  [unwired: 3 in, 1 out]
            n33 = for {
              tunnel: w71 -> [w84] mode=indexing
              tunnel: [w83] -> w64 mode=indexing
              # "s"
              # "h"
              # "m"
              # "s"
              # "ms"
              n34 = call <vilib>:"Trim Whitespace.vi"("string"=w84) -> ("trimmed string"=w95:string)  [unwired: 1 in]
              n35 = String Length(string=w95) -> (length=w96:i32)
              n36 = case shown="..9, 기본" w96 {
                tunnel: w95 -> [w107 w111]
                tunnel: [w102 w114] -> w89
                tunnel: [w101 w115] -> w88
                tunnel: [w100 w116] -> w85
                tunnel: [0 ("인덱스") w109] -> w90
                frame ..9, Default {
                  # "분:초.000"
                  n37 = Scan From String(format string="%02d" ("포맷 문자열"), input string=w107) -> (remaining string=w104:string, output 1=w102:i32)  [unwired: 3 in, 2 out]
                  n38 = Scan From String(format string="%02d" ("포맷 문자열"), input string=w104, initial scan location=u32 1 ("초기 스캔 위치")) -> (remaining string=w103:string, output 1=w101:i32)  [unwired: 2 in, 2 out]
                  n39 = Scan From String(format string="%03d" ("포맷 문자열"), input string=w103, initial scan location=u32 1 ("초기 스캔 위치")) -> (output 1=w100:i32)  [unwired: 2 in, 3 out]
                }
                frame 10.. {
                  # "시:분:초.000"
                  n40 = Scan From String(format string="%02d" ("포맷 문자열"), input string=w111) -> (remaining string=w110:string, output 1=w109:i32)  [unwired: 3 in, 2 out]
                  n41 = Scan From String(format string="%02d" ("포맷 문자열"), input string=w110, initial scan location=u32 1 ("초기 스캔 위치")) -> (remaining string=w120:string, output 1=w114:i32)  [unwired: 2 in, 2 out]
                  n42 = Scan From String(format string="%02d" ("포맷 문자열"), input string=w120, initial scan location=u32 1 ("초기 스캔 위치")) -> (remaining string=w119:string, output 1=w115:i32)  [unwired: 2 in, 2 out]
                  n43 = Scan From String(format string="%03d" ("포맷 문자열"), input string=w119, initial scan location=u32 1 ("초기 스캔 위치")) -> (output 1=w116:i32)  [unwired: 2 in, 3 out]
                }
              }
              n44 = Multiply(x=w90, y=3600.0) -> (x*y=w92:dbl)
              n45 = Multiply(x=w85, y=0.001) -> (x*y=w86:dbl)
              n46 = Multiply(x=w89, y=60.0) -> (x*y=w91:dbl)
              n47 = Compound Arithmetic op=ADD(w92, w91, w88, w86) -> (w83:dbl)
            }
            n48 = Array Size(array=w58) -> (size(s)=→"Data Length":i32)
            n49 = Array Max & Min(array=w58) -> (max value=w61:dbl, min value=w31:dbl)  [unwired: 2 out]
            n50 = Array Max & Min(array=w47) -> (max value=w52:dbl, min value=w27:dbl)  [unwired: 2 out]
            n51 = Subtract(x=w61, y=w31) -> (x-y=w32:dbl)
            n52 = Subtract(x=w52, y=w27) -> (x-y=w26:dbl)
            n53 = Multiply(x=w32, y=w25) -> (x*y=w30:dbl)
            n54 = Multiply(x=w26, y=w25) -> (x*y=w28:dbl)
            n55 = Add(x=w31, y=w30) -> (x+y=w29:dbl)
            n56 = Add(x=w27, y=w28) -> (x+y=w24:dbl)
            n57 = Subtract(x=w61, y=w31) -> (x-y=w38:dbl)
            "Delta-Raw" <- w38
            n58 = Subtract(x=w52, y=w27) -> (x-y=w36:dbl)
            "Delta-Filter" <- w36
            n59 = Multiply(x=w38, y="hysteresis") -> (x*y=w37:dbl)
            n60 = Multiply(x=w36, y="hysteresis") -> (x*y=w35:dbl)
            n61 = call-poly <vilib>:"Basic Level Trigger Detection.vi"("signal in"=w58, "level"=w29, "hysteresis"=w37, "location mode"=w59, "trigger slope"=w60) -> ("trigger location"=w57:dbl, "trigger detected?"=→"trigger detected?":bool)  [unwired: 8 in, 1 out]
            n62 = call-poly <vilib>:"Basic Level Trigger Detection.vi"("signal in"=w47, "level"=w24, "hysteresis"=w35, "location mode"=w54, "trigger slope"=w53) -> ("trigger location"=w49:dbl, "trigger detected?"=→"trigger detected? 2":bool)  [unwired: 8 in, 1 out]
            n63 = Index Array(array=w58, index=w57) -> (element=w55:dbl)
            n64 = Index Array(array=w47, index=w49) -> (element=w51:dbl)
            n65 = Index Array(array=w64, index=0 ("인덱스")) -> (element=w63:dbl)
            n66 = Subtract(x=w64, y=w63) -> (x-y=w48:dbl[])
            n67 = Bundle(w48, w47) -> (w67:cluster{dbl[], dbl[]})  [unwired: 1 in]
            n68 = Bundle(w48, w58) -> (w68:cluster{dbl[], dbl[]})  [unwired: 1 in]
            n69 = Index Array(array=w48, index=w57) -> (element=w46:dbl)
            n70 = Index Array(array=w48, index=w49) -> (element=w45:dbl)
            n71 = Build Array(w46, w45) -> (w42:dbl[])
            n72 = Array Max & Min(array=w42) -> (max value=w43:dbl, min value=w44:dbl)  [unwired: 2 out]
            n73 = property on="Response Time Graph" class="XYGraph (엄격한)"("Active Cursor"=u32 0 ("활성 커서"), "Cursor.Cursor X"=w46, "Cursor.Cursor Y"=w55) -> ()  [unwired: 2 in, 2 out]
            n74 = property on="Response Time Graph" class="XYGraph (엄격한)"("Active Cursor"=u32 1 ("활성 커서"), "Cursor.Cursor X"=w45, "Cursor.Cursor Y"=w51) -> ()  [unwired: 2 in, 2 out]
            n75 = Build Array(w68, w67) -> (→"Response Time Graph":cluster{dbl[], dbl[]}[])
            n76 = Subtract(x=w43, y=w44) -> (x-y=→"Delay_time(s)":dbl)
          }
          frame #3 {
            n77 = property on="Response Time Graph" class="XYGraph (엄격한)"("Active Cursor"=u32 0 ("활성 커서")) -> ("Cursor.Cursor X"=w129:dbl, "Cursor.Cursor Y"=w127:dbl)  [unwired: 2 in, 2 out]
            n78 = property on="Response Time Graph" class="XYGraph (엄격한)"("Active Cursor"=u32 1 ("활성 커서")) -> ("Cursor.Cursor X"=w125:dbl, "Cursor.Cursor Y"=w124:dbl)  [unwired: 2 in, 2 out]
            n79 = Format Into String(format string="[cursor_raw]\n X: %.3f,  Y: %.7f\n\n[cursor_filter]\n X: %.3f,  Y: %.7f" ("포맷 문자열"), w129, w127, w125, w124) -> (resulting string=w128:string)  [unwired: 2 in, 1 out]
            n80 = local write "Cursor Info."(w128) -> ()
            n81 = local write "Calcuration"(FALSE ("Calcuration")) -> ()
          }
        }
      }
    }
    n82 = Wait Until Next ms Multiple(millisecond multiple=u32 100 ("ms 배수")) -> ()  [unwired: 1 out]
    n83 = local read "Exit"() -> (w12:bool)
  }
